vi "Link Control References.vi"(8 "error in":errorcluster, 10 "Control Map":T1[](array[typedef]), 11 "DIG_IO in":refnum<class "DIG_IO.lvclass">) -> (0 "error out":errorcluster, 3 "DIG_IO out":refnum<class "DIG_IO.lvclass">)   [LabVIEW 2019, in "DIG_IO.lvlib" / "DIG_IO.lvclass"]
uses:
  Library/DIG_IO.lvclass
  builds/Instruments/Instruments.lvlibp/Custom Controls/Control Element.ctl
  Library/DIG_IO.lvclass/DIG_IO.ctl
  builds/Instruments/Instruments.lvlibp/Library/Instruments.lvclass
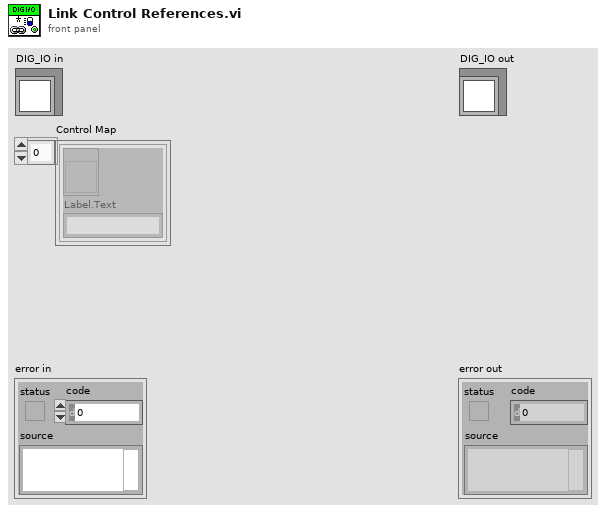
[diagram p1: front panel]
types:
  T1 = typedef "Instruments.lvlibp/Instruments.lvclass/Control Element.ctl" = cluster{refnum<vi>, "Label.Text":string}
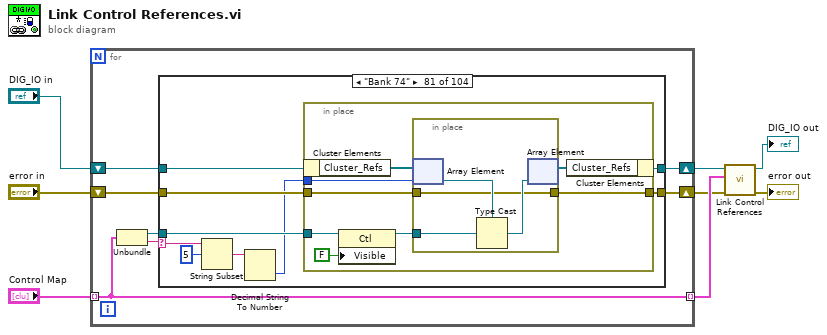
[diagram p0: block diagram]
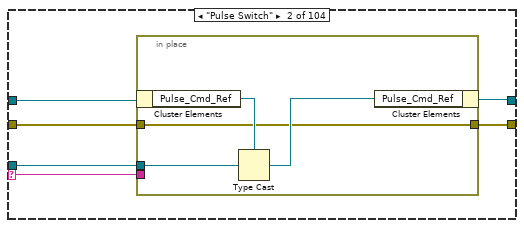
[diagram p3: hidden frame]
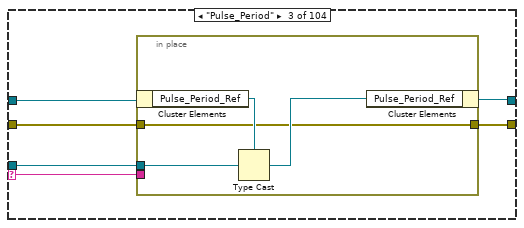
[diagram p4: hidden frame]
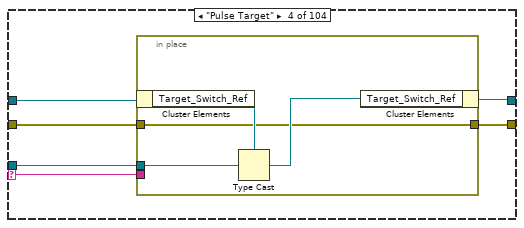
[diagram p5: hidden frame]
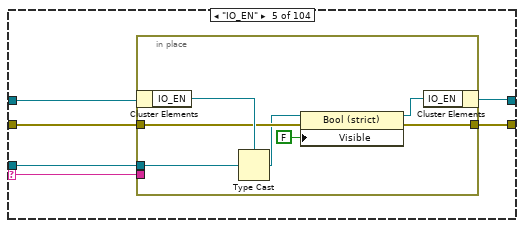
[diagram p6: hidden frame]
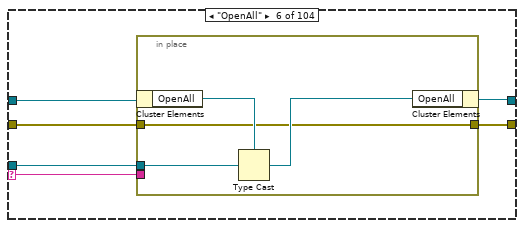
[diagram p7: hidden frame]
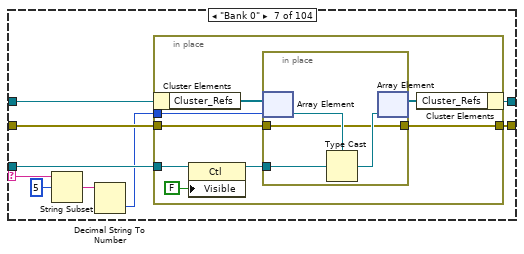
[diagram p8: hidden frame]
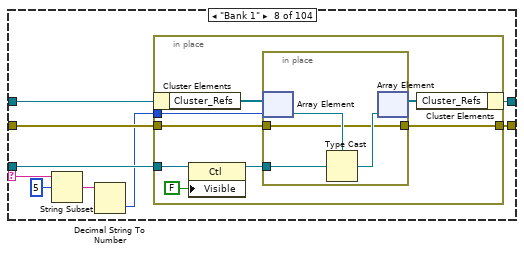
[diagram p9: hidden frame]
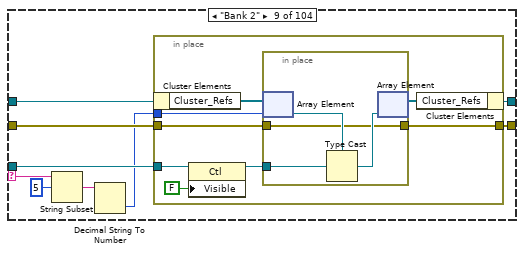
[diagram p10: hidden frame]
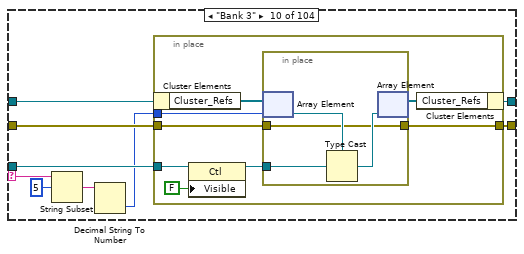
[diagram p11: hidden frame]
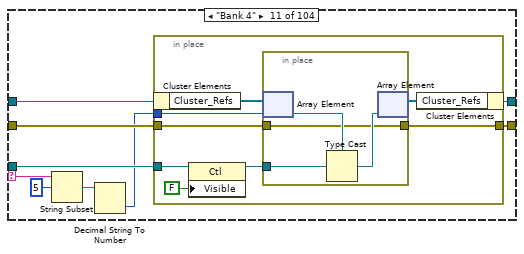
[diagram p12: hidden frame]
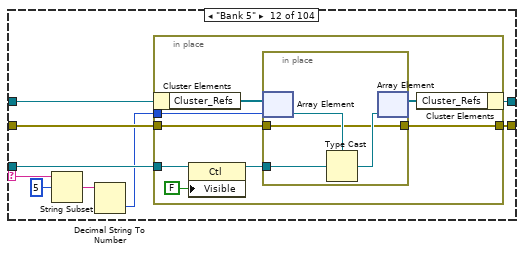
[diagram p13: hidden frame]
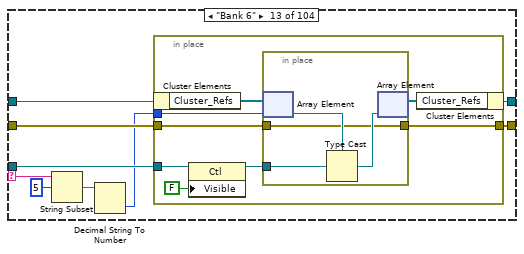
[diagram p14: hidden frame]
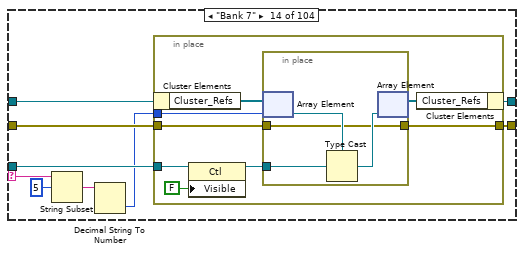
[diagram p15: hidden frame]
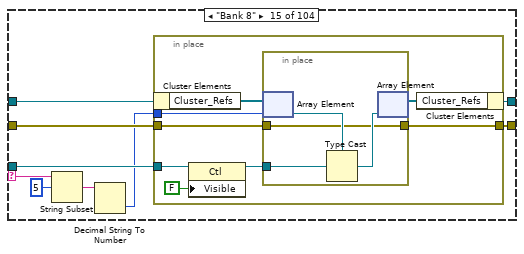
[diagram p16: hidden frame]
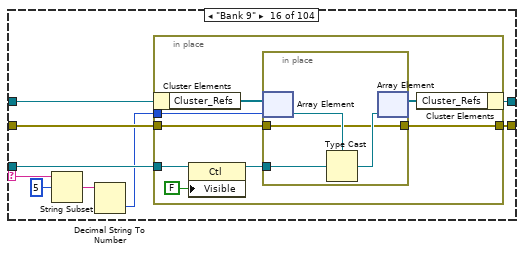
[diagram p17: hidden frame]
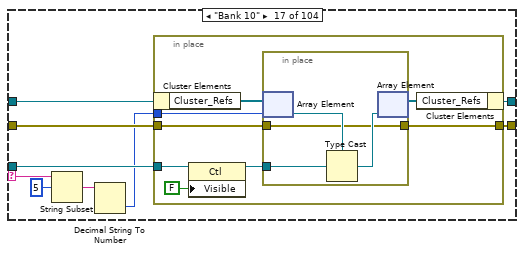
[diagram p18: hidden frame]
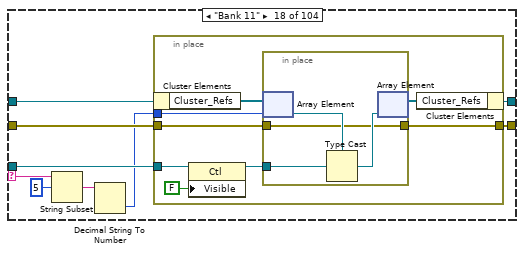
[diagram p19: hidden frame]
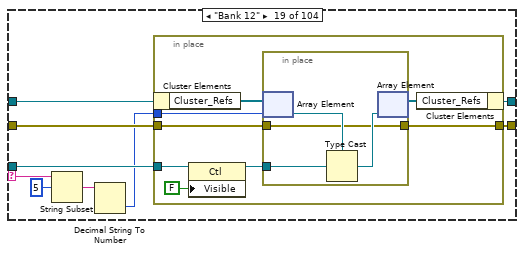
[diagram p20: hidden frame]
diagram:
  n1 = for {
    tunnel: "Control Map" -> [w15] mode=indexing
    tunnel: [w15] -> w5 mode=indexing
    shift-right: [w9] -> w3
    shift-left: "error in" -> [w12]
    shift-right: [w10] -> w1
    shift-left: "DIG_IO in" -> [w11]
    n2 = Unbundle(w15) -> (w13:refnum<vi>, "Label.Text"=w14:string)
    n3 = case shown="\"Bank 74\"" w14 {
      selector: w14 -> [_ w19 w29 w39 w49 w62 w72 w93 w114 w135 w156 w177 w198 w219 w240 w261 w282 w303 w324 w345 w366 w387 w408 w429 w450 w471 w492 w513 w534 w555 w576 w597 w618 w639 w660 w681 w702 w723 w744 w765 w786 w807 w828 w849 w870 w891 w912 w933 w954 w975 w996 w1017 w1038 w1059 w1080 w1101 w1122 w1143 w1164 w1185 w1206 w1227 w1248 w1269 w1290 w1311 w1332 w1353 w1374 w1395 w1416 w1437 w1458 w1479 w1500 w1521 w1542 w1563 w1584 w1605 w1626 w1647 w1668 w1689 w1710 w1731 w1752 w1773 w1794 w1815 w1836 w1857 w1878 w1899 w1920 w1941 w1962 w1983 w2004 w2025 w2046 w2067 w2088 w2103]
      tunnel: w13 -> [_ w20 w30 w40 w50 w63 w76 w97 w118 w139 w160 w181 w202 w223 w244 w265 w286 w307 w328 w349 w370 w391 w412 w433 w454 w475 w496 w517 w538 w559 w580 w601 w622 w643 w664 w685 w706 w727 w748 w769 w790 w811 w832 w853 w874 w895 w916 w937 w958 w979 w1000 w1021 w1042 w1063 w1084 w1105 w1126 w1147 w1168 w1189 w1210 w1231 w1252 w1273 w1294 w1315 w1336 w1357 w1378 w1399 w1420 w1441 w1462 w1483 w1504 w1525 w1546 w1567 w1588 w1609 w1630 w1651 w1672 w1693 w1714 w1735 w1756 w1777 w1798 w1819 w1840 w1861 w1882 w1903 w1924 w1945 w1966 w1987 w2008 w2029 w2050 w2071 w2092 w2107]
      tunnel: w12 -> [w16 w22 w32 w42 w52 w65 w78 w99 w120 w141 w162 w183 w204 w225 w246 w267 w288 w309 w330 w351 w372 w393 w414 w435 w456 w477 w498 w519 w540 w561 w582 w603 w624 w645 w666 w687 w708 w729 w750 w771 w792 w813 w834 w855 w876 w897 w918 w939 w960 w981 w1002 w1023 w1044 w1065 w1086 w1107 w1128 w1149 w1170 w1191 w1212 w1233 w1254 w1275 w1296 w1317 w1338 w1359 w1380 w1401 w1422 w1443 w1464 w1485 w1506 w1527 w1548 w1569 w1590 w1611 w1632 w1653 w1674 w1695 w1716 w1737 w1758 w1779 w1800 w1821 w1842 w1863 w1884 w1905 w1926 w1947 w1968 w1989 w2010 w2031 w2052 w2073 w2094 w2109]
      tunnel: w11 -> [w17 w23 w33 w43 w53 w66 w79 w100 w121 w142 w163 w184 w205 w226 w247 w268 w289 w310 w331 w352 w373 w394 w415 w436 w457 w478 w499 w520 w541 w562 w583 w604 w625 w646 w667 w688 w709 w730 w751 w772 w793 w814 w835 w856 w877 w898 w919 w940 w961 w982 w1003 w1024 w1045 w1066 w1087 w1108 w1129 w1150 w1171 w1192 w1213 w1234 w1255 w1276 w1297 w1318 w1339 w1360 w1381 w1402 w1423 w1444 w1465 w1486 w1507 w1528 w1549 w1570 w1591 w1612 w1633 w1654 w1675 w1696 w1717 w1738 w1759 w1780 w1801 w1822 w1843 w1864 w1885 w1906 w1927 w1948 w1969 w1990 w2011 w2032 w2053 w2074 w2095 w2110]
      tunnel: [w17 w21 w31 w41 w51 w64 w77 w98 w119 w140 w161 w182 w203 w224 w245 w266 w287 w308 w329 w350 w371 w392 w413 w434 w455 w476 w497 w518 w539 w560 w581 w602 w623 w644 w665 w686 w707 w728 w749 w770 w791 w812 w833 w854 w875 w896 w917 w938 w959 w980 w1001 w1022 w1043 w1064 w1085 w1106 w1127 w1148 w1169 w1190 w1211 w1232 w1253 w1274 w1295 w1316 w1337 w1358 w1379 w1400 w1421 w1442 w1463 w1484 w1505 w1526 w1547 w1568 w1589 w1610 w1631 w1652 w1673 w1694 w1715 w1736 w1757 w1778 w1799 w1820 w1841 w1862 w1883 w1904 w1925 w1946 w1967 w1988 w2009 w2030 w2051 w2072 w2093 w2108] -> w10
      tunnel: [w16 w18 w28 w38 w48 w61 w75 w96 w117 w138 w159 w180 w201 w222 w243 w264 w285 w306 w327 w348 w369 w390 w411 w432 w453 w474 w495 w516 w537 w558 w579 w600 w621 w642 w663 w684 w705 w726 w747 w768 w789 w810 w831 w852 w873 w894 w915 w936 w957 w978 w999 w1020 w1041 w1062 w1083 w1104 w1125 w1146 w1167 w1188 w1209 w1230 w1251 w1272 w1293 w1314 w1335 w1356 w1377 w1398 w1419 w1440 w1461 w1482 w1503 w1524 w1545 w1566 w1587 w1608 w1629 w1650 w1671 w1692 w1713 w1734 w1755 w1776 w1797 w1818 w1839 w1860 w1881 w1902 w1923 w1944 w1965 w1986 w2007 w2028 w2049 w2070 w2091 w2106] -> w9
      frame Default {
      }
      frame "Pulse Switch" {
        n4 = in-place {
          in-place-border: w22 -> [w24]
          in-place-border: w20 -> [w26]
          in-place-border: w19 -> [_]
          in-place-border: [w24] -> w18
          n5 = in-place-cluster #1(w23) -> ("Pulse_Cmd_Ref"=w27:refnum<vi>)
          n6 = Type Cast(type=w27, x=w26) -> (*(type *) &x=w25:refnum<vi>)
          n7 = in-place-cluster #1("Pulse_Cmd_Ref"=w25) -> (w21:refnum<class "DIG_IO.lvclass">)
        }
      }
      frame "Pulse_Period" {
        n8 = in-place {
          in-place-border: w32 -> [w34]
          in-place-border: w30 -> [w36]
          in-place-border: w29 -> [_]
          in-place-border: [w34] -> w28
          n9 = in-place-cluster #2(w33) -> ("Pulse_Period_Ref"=w37:refnum<vi>)
          n10 = Type Cast(type=w37, x=w36) -> (*(type *) &x=w35:refnum<vi>)
          n11 = in-place-cluster #2("Pulse_Period_Ref"=w35) -> (w31:refnum<class "DIG_IO.lvclass">)
        }
      }
      frame "Pulse Target" {
        n12 = in-place {
          in-place-border: w42 -> [w44]
          in-place-border: w40 -> [w46]
          in-place-border: w39 -> [_]
          in-place-border: [w44] -> w38
          n13 = in-place-cluster #3(w43) -> ("Target_Switch_Ref"=w47:refnum<vi>)
          n14 = Type Cast(type=w47, x=w46) -> (*(type *) &x=w45:refnum<vi>)
          n15 = in-place-cluster #3("Target_Switch_Ref"=w45) -> (w41:refnum<class "DIG_IO.lvclass">)
        }
      }
      frame "IO_EN" {
        n16 = in-place {
          in-place-border: w52 -> [w58]
          in-place-border: w50 -> [w59]
          in-place-border: w49 -> [_]
          in-place-border: [w57] -> w48
          n17 = in-place-cluster #4(w53) -> ("IO_EN"=w60:refnum<vi>)
          n18 = Type Cast(type=w60, x=w59) -> (*(type *) &x=w56:refnum<vi>)
          n19 = property class="Bool (strict)"(reference=w56, error in=w58, "Visible"=FALSE) -> (reference out=w55:refnum<vi>, error out=w57:errorcluster)
          n20 = in-place-cluster #4("IO_EN"=w55) -> (w51:refnum<class "DIG_IO.lvclass">)
        }
      }
      frame "OpenAll" {
        n21 = in-place {
          in-place-border: w65 -> [w67]
          in-place-border: w63 -> [w69]
          in-place-border: w62 -> [_]
          in-place-border: [w67] -> w61
          n22 = in-place-cluster #5(w66) -> ("OpenAll"=w70:refnum<vi>)
          n23 = Type Cast(type=w70, x=w69) -> (*(type *) &x=w68:refnum<vi>)
          n24 = in-place-cluster #5("OpenAll"=w68) -> (w64:refnum<class "DIG_IO.lvclass">)
        }
      }
      frame "Bank 0" {
        n25 = String Subset(string=w72, offset (0)=5) -> (substring=w74:string)  [unwired: 1 in]
        n26 = Decimal String To Number(string=w74) -> (number=w71:i32)  [unwired: 2 in, 1 out]
        n27 = in-place {
          in-place-border: w78 -> [w84]
          in-place-border: w76 -> [w85]
          in-place-border: [w83] -> w75
          in-place-border: w71 -> [w82]
          n28 = in-place-cluster #6(w79) -> ("Cluster_Refs"=w87:refnum<vi>[])
          n29 = property class="Ctl"(reference=w85, "Visible"=FALSE) -> (reference out=w81:refnum<vi>)  [unwired: 1 in, 1 out]
          n30 = in-place {
            in-place-border: w81 -> [w90]
            in-place-border: w84 -> [w88]
            in-place-border: [w88] -> w83
            n31 = in-place-array #7(w87, w82) -> (w91:refnum<vi>)
            n32 = Type Cast(type=w91, x=w90) -> (*(type *) &x=w89:refnum<vi>)
            n33 = in-place-array #7(w89) -> (w86:refnum<vi>[])  [unwired: 1 out]
          }
          n34 = in-place-cluster #6("Cluster_Refs"=w86) -> (w77:refnum<class "DIG_IO.lvclass">)
        }
      }
      frame "Bank 1" {
        n35 = String Subset(string=w93, offset (0)=5) -> (substring=w95:string)  [unwired: 1 in]
        n36 = Decimal String To Number(string=w95) -> (number=w92:i32)  [unwired: 2 in, 1 out]
        n37 = in-place {
          in-place-border: w99 -> [w105]
          in-place-border: w97 -> [w106]
          in-place-border: [w104] -> w96
          in-place-border: w92 -> [w103]
          n38 = in-place-cluster #8(w100) -> ("Cluster_Refs"=w108:refnum<vi>[])
          n39 = property class="Ctl"(reference=w106, "Visible"=FALSE) -> (reference out=w102:refnum<vi>)  [unwired: 1 in, 1 out]
          n40 = in-place {
            in-place-border: w102 -> [w111]
            in-place-border: w105 -> [w109]
            in-place-border: [w109] -> w104
            n41 = in-place-array #9(w108, w103) -> (w112:refnum<vi>)
            n42 = Type Cast(type=w112, x=w111) -> (*(type *) &x=w110:refnum<vi>)
            n43 = in-place-array #9(w110) -> (w107:refnum<vi>[])  [unwired: 1 out]
          }
          n44 = in-place-cluster #8("Cluster_Refs"=w107) -> (w98:refnum<class "DIG_IO.lvclass">)
        }
      }
      frame "Bank 2" {
        n45 = String Subset(string=w114, offset (0)=5) -> (substring=w116:string)  [unwired: 1 in]
        n46 = Decimal String To Number(string=w116) -> (number=w113:i32)  [unwired: 2 in, 1 out]
        n47 = in-place {
          in-place-border: w120 -> [w126]
          in-place-border: w118 -> [w127]
          in-place-border: [w125] -> w117
          in-place-border: w113 -> [w124]
          n48 = in-place-cluster #10(w121) -> ("Cluster_Refs"=w129:refnum<vi>[])
          n49 = property class="Ctl"(reference=w127, "Visible"=FALSE) -> (reference out=w123:refnum<vi>)  [unwired: 1 in, 1 out]
          n50 = in-place {
            in-place-border: w123 -> [w132]
            in-place-border: w126 -> [w130]
            in-place-border: [w130] -> w125
            n51 = in-place-array #11(w129, w124) -> (w133:refnum<vi>)
            n52 = Type Cast(type=w133, x=w132) -> (*(type *) &x=w131:refnum<vi>)
            n53 = in-place-array #11(w131) -> (w128:refnum<vi>[])  [unwired: 1 out]
          }
          n54 = in-place-cluster #10("Cluster_Refs"=w128) -> (w119:refnum<class "DIG_IO.lvclass">)
        }
      }
      frame "Bank 3" {
        n55 = String Subset(string=w135, offset (0)=5) -> (substring=w137:string)  [unwired: 1 in]
        n56 = Decimal String To Number(string=w137) -> (number=w134:i32)  [unwired: 2 in, 1 out]
        n57 = in-place {
          in-place-border: w141 -> [w147]
          in-place-border: w139 -> [w148]
          in-place-border: [w146] -> w138
          in-place-border: w134 -> [w145]
          n58 = in-place-cluster #12(w142) -> ("Cluster_Refs"=w150:refnum<vi>[])
          n59 = property class="Ctl"(reference=w148, "Visible"=FALSE) -> (reference out=w144:refnum<vi>)  [unwired: 1 in, 1 out]
          n60 = in-place {
            in-place-border: w144 -> [w153]
            in-place-border: w147 -> [w151]
            in-place-border: [w151] -> w146
            n61 = in-place-array #13(w150, w145) -> (w154:refnum<vi>)
            n62 = Type Cast(type=w154, x=w153) -> (*(type *) &x=w152:refnum<vi>)
            n63 = in-place-array #13(w152) -> (w149:refnum<vi>[])  [unwired: 1 out]
          }
          n64 = in-place-cluster #12("Cluster_Refs"=w149) -> (w140:refnum<class "DIG_IO.lvclass">)
        }
      }
      frame "Bank 4" {
        n65 = String Subset(string=w156, offset (0)=5) -> (substring=w158:string)  [unwired: 1 in]
        n66 = Decimal String To Number(string=w158) -> (number=w155:i32)  [unwired: 2 in, 1 out]
        n67 = in-place {
          in-place-border: w162 -> [w168]
          in-place-border: w160 -> [w169]
          in-place-border: [w167] -> w159
          in-place-border: w155 -> [w166]
          n68 = in-place-cluster #14(w163) -> ("Cluster_Refs"=w171:refnum<vi>[])
          n69 = property class="Ctl"(reference=w169, "Visible"=FALSE) -> (reference out=w165:refnum<vi>)  [unwired: 1 in, 1 out]
          n70 = in-place {
            in-place-border: w165 -> [w174]
            in-place-border: w168 -> [w172]
            in-place-border: [w172] -> w167
            n71 = in-place-array #15(w171, w166) -> (w175:refnum<vi>)
            n72 = Type Cast(type=w175, x=w174) -> (*(type *) &x=w173:refnum<vi>)
            n73 = in-place-array #15(w173) -> (w170:refnum<vi>[])  [unwired: 1 out]
          }
          n74 = in-place-cluster #14("Cluster_Refs"=w170) -> (w161:refnum<class "DIG_IO.lvclass">)
        }
      }
      frame "Bank 5" {
        n75 = String Subset(string=w177, offset (0)=5) -> (substring=w179:string)  [unwired: 1 in]
        n76 = Decimal String To Number(string=w179) -> (number=w176:i32)  [unwired: 2 in, 1 out]
        n77 = in-place {
          in-place-border: w183 -> [w189]
          in-place-border: w181 -> [w190]
          in-place-border: [w188] -> w180
          in-place-border: w176 -> [w187]
          n78 = in-place-cluster #16(w184) -> ("Cluster_Refs"=w192:refnum<vi>[])
          n79 = property class="Ctl"(reference=w190, "Visible"=FALSE) -> (reference out=w186:refnum<vi>)  [unwired: 1 in, 1 out]
          n80 = in-place {
            in-place-border: w186 -> [w195]
            in-place-border: w189 -> [w193]
            in-place-border: [w193] -> w188
            n81 = in-place-array #17(w192, w187) -> (w196:refnum<vi>)
            n82 = Type Cast(type=w196, x=w195) -> (*(type *) &x=w194:refnum<vi>)
            n83 = in-place-array #17(w194) -> (w191:refnum<vi>[])  [unwired: 1 out]
          }
          n84 = in-place-cluster #16("Cluster_Refs"=w191) -> (w182:refnum<class "DIG_IO.lvclass">)
        }
      }
      frame "Bank 6" {
        n85 = String Subset(string=w198, offset (0)=5) -> (substring=w200:string)  [unwired: 1 in]
        n86 = Decimal String To Number(string=w200) -> (number=w197:i32)  [unwired: 2 in, 1 out]
        n87 = in-place {
          in-place-border: w204 -> [w210]
          in-place-border: w202 -> [w211]
          in-place-border: [w209] -> w201
          in-place-border: w197 -> [w208]
          n88 = in-place-cluster #18(w205) -> ("Cluster_Refs"=w213:refnum<vi>[])
          n89 = property class="Ctl"(reference=w211, "Visible"=FALSE) -> (reference out=w207:refnum<vi>)  [unwired: 1 in, 1 out]
          n90 = in-place {
            in-place-border: w207 -> [w216]
            in-place-border: w210 -> [w214]
            in-place-border: [w214] -> w209
            n91 = in-place-array #19(w213, w208) -> (w217:refnum<vi>)
            n92 = Type Cast(type=w217, x=w216) -> (*(type *) &x=w215:refnum<vi>)
            n93 = in-place-array #19(w215) -> (w212:refnum<vi>[])  [unwired: 1 out]
          }
          n94 = in-place-cluster #18("Cluster_Refs"=w212) -> (w203:refnum<class "DIG_IO.lvclass">)
        }
      }
      frame "Bank 7" {
        n95 = String Subset(string=w219, offset (0)=5) -> (substring=w221:string)  [unwired: 1 in]
        n96 = Decimal String To Number(string=w221) -> (number=w218:i32)  [unwired: 2 in, 1 out]
        n97 = in-place {
          in-place-border: w225 -> [w231]
          in-place-border: w223 -> [w232]
          in-place-border: [w230] -> w222
          in-place-border: w218 -> [w229]
          n98 = in-place-cluster #20(w226) -> ("Cluster_Refs"=w234:refnum<vi>[])
          n99 = property class="Ctl"(reference=w232, "Visible"=FALSE) -> (reference out=w228:refnum<vi>)  [unwired: 1 in, 1 out]
          n100 = in-place {
            in-place-border: w228 -> [w237]
            in-place-border: w231 -> [w235]
            in-place-border: [w235] -> w230
            n101 = in-place-array #21(w234, w229) -> (w238:refnum<vi>)
            n102 = Type Cast(type=w238, x=w237) -> (*(type *) &x=w236:refnum<vi>)
            n103 = in-place-array #21(w236) -> (w233:refnum<vi>[])  [unwired: 1 out]
          }
          n104 = in-place-cluster #20("Cluster_Refs"=w233) -> (w224:refnum<class "DIG_IO.lvclass">)
        }
      }
      frame "Bank 8" {
        n105 = String Subset(string=w240, offset (0)=5) -> (substring=w242:string)  [unwired: 1 in]
        n106 = Decimal String To Number(string=w242) -> (number=w239:i32)  [unwired: 2 in, 1 out]
        n107 = in-place {
          in-place-border: w246 -> [w252]
          in-place-border: w244 -> [w253]
          in-place-border: [w251] -> w243
          in-place-border: w239 -> [w250]
          n108 = in-place-cluster #22(w247) -> ("Cluster_Refs"=w255:refnum<vi>[])
          n109 = property class="Ctl"(reference=w253, "Visible"=FALSE) -> (reference out=w249:refnum<vi>)  [unwired: 1 in, 1 out]
          n110 = in-place {
            in-place-border: w249 -> [w258]
            in-place-border: w252 -> [w256]
            in-place-border: [w256] -> w251
            n111 = in-place-array #23(w255, w250) -> (w259:refnum<vi>)
            n112 = Type Cast(type=w259, x=w258) -> (*(type *) &x=w257:refnum<vi>)
            n113 = in-place-array #23(w257) -> (w254:refnum<vi>[])  [unwired: 1 out]
          }
          n114 = in-place-cluster #22("Cluster_Refs"=w254) -> (w245:refnum<class "DIG_IO.lvclass">)
        }
      }
      frame "Bank 9" {
        n115 = String Subset(string=w261, offset (0)=5) -> (substring=w263:string)  [unwired: 1 in]
        n116 = Decimal String To Number(string=w263) -> (number=w260:i32)  [unwired: 2 in, 1 out]
        n117 = in-place {
          in-place-border: w267 -> [w273]
          in-place-border: w265 -> [w274]
          in-place-border: [w272] -> w264
          in-place-border: w260 -> [w271]
          n118 = in-place-cluster #24(w268) -> ("Cluster_Refs"=w276:refnum<vi>[])
          n119 = property class="Ctl"(reference=w274, "Visible"=FALSE) -> (reference out=w270:refnum<vi>)  [unwired: 1 in, 1 out]
          n120 = in-place {
            in-place-border: w270 -> [w279]
            in-place-border: w273 -> [w277]
            in-place-border: [w277] -> w272
            n121 = in-place-array #25(w276, w271) -> (w280:refnum<vi>)
            n122 = Type Cast(type=w280, x=w279) -> (*(type *) &x=w278:refnum<vi>)
            n123 = in-place-array #25(w278) -> (w275:refnum<vi>[])  [unwired: 1 out]
          }
          n124 = in-place-cluster #24("Cluster_Refs"=w275) -> (w266:refnum<class "DIG_IO.lvclass">)
        }
      }
      frame "Bank 10" {
        n125 = String Subset(string=w282, offset (0)=5) -> (substring=w284:string)  [unwired: 1 in]
        n126 = Decimal String To Number(string=w284) -> (number=w281:i32)  [unwired: 2 in, 1 out]
        n127 = in-place {
          in-place-border: w288 -> [w294]
          in-place-border: w286 -> [w295]
          in-place-border: [w293] -> w285
          in-place-border: w281 -> [w292]
          n128 = in-place-cluster #26(w289) -> ("Cluster_Refs"=w297:refnum<vi>[])
          n129 = property class="Ctl"(reference=w295, "Visible"=FALSE) -> (reference out=w291:refnum<vi>)  [unwired: 1 in, 1 out]
          n130 = in-place {
            in-place-border: w291 -> [w300]
            in-place-border: w294 -> [w298]
            in-place-border: [w298] -> w293
            n131 = in-place-array #27(w297, w292) -> (w301:refnum<vi>)
            n132 = Type Cast(type=w301, x=w300) -> (*(type *) &x=w299:refnum<vi>)
            n133 = in-place-array #27(w299) -> (w296:refnum<vi>[])  [unwired: 1 out]
          }
          n134 = in-place-cluster #26("Cluster_Refs"=w296) -> (w287:refnum<class "DIG_IO.lvclass">)
        }
      }
      frame "Bank 11" {
        n135 = String Subset(string=w303, offset (0)=5) -> (substring=w305:string)  [unwired: 1 in]
        n136 = Decimal String To Number(string=w305) -> (number=w302:i32)  [unwired: 2 in, 1 out]
        n137 = in-place {
          in-place-border: w309 -> [w315]
          in-place-border: w307 -> [w316]
          in-place-border: [w314] -> w306
          in-place-border: w302 -> [w313]
          n138 = in-place-cluster #28(w310) -> ("Cluster_Refs"=w318:refnum<vi>[])
          n139 = property class="Ctl"(reference=w316, "Visible"=FALSE) -> (reference out=w312:refnum<vi>)  [unwired: 1 in, 1 out]
          n140 = in-place {
            in-place-border: w312 -> [w321]
            in-place-border: w315 -> [w319]
            in-place-border: [w319] -> w314
            n141 = in-place-array #29(w318, w313) -> (w322:refnum<vi>)
            n142 = Type Cast(type=w322, x=w321) -> (*(type *) &x=w320:refnum<vi>)
            n143 = in-place-array #29(w320) -> (w317:refnum<vi>[])  [unwired: 1 out]
          }
          n144 = in-place-cluster #28("Cluster_Refs"=w317) -> (w308:refnum<class "DIG_IO.lvclass">)
        }
      }
      frame "Bank 12" {
        n145 = String Subset(string=w324, offset (0)=5) -> (substring=w326:string)  [unwired: 1 in]
        n146 = Decimal String To Number(string=w326) -> (number=w323:i32)  [unwired: 2 in, 1 out]
        n147 = in-place {
          in-place-border: w330 -> [w336]
          in-place-border: w328 -> [w337]
          in-place-border: [w335] -> w327
          in-place-border: w323 -> [w334]
          n148 = in-place-cluster #30(w331) -> ("Cluster_Refs"=w339:refnum<vi>[])
          n149 = property class="Ctl"(reference=w337, "Visible"=FALSE) -> (reference out=w333:refnum<vi>)  [unwired: 1 in, 1 out]
          n150 = in-place {
            in-place-border: w333 -> [w342]
            in-place-border: w336 -> [w340]
            in-place-border: [w340] -> w335
            n151 = in-place-array #31(w339, w334) -> (w343:refnum<vi>)
            n152 = Type Cast(type=w343, x=w342) -> (*(type *) &x=w341:refnum<vi>)
            n153 = in-place-array #31(w341) -> (w338:refnum<vi>[])  [unwired: 1 out]
          }
          n154 = in-place-cluster #30("Cluster_Refs"=w338) -> (w329:refnum<class "DIG_IO.lvclass">)
        }
      }
      frame "Bank 13" {
        n155 = String Subset(string=w345, offset (0)=5) -> (substring=w347:string)  [unwired: 1 in]
        n156 = Decimal String To Number(string=w347) -> (number=w344:i32)  [unwired: 2 in, 1 out]
        n157 = in-place {
          in-place-border: w351 -> [w357]
          in-place-border: w349 -> [w358]
          in-place-border: [w356] -> w348
          in-place-border: w344 -> [w355]
          n158 = in-place-cluster #32(w352) -> ("Cluster_Refs"=w360:refnum<vi>[])
          n159 = property class="Ctl"(reference=w358, "Visible"=FALSE) -> (reference out=w354:refnum<vi>)  [unwired: 1 in, 1 out]
          n160 = in-place {
            in-place-border: w354 -> [w363]
            in-place-border: w357 -> [w361]
            in-place-border: [w361] -> w356
            n161 = in-place-array #33(w360, w355) -> (w364:refnum<vi>)
            n162 = Type Cast(type=w364, x=w363) -> (*(type *) &x=w362:refnum<vi>)
            n163 = in-place-array #33(w362) -> (w359:refnum<vi>[])  [unwired: 1 out]
          }
          n164 = in-place-cluster #32("Cluster_Refs"=w359) -> (w350:refnum<class "DIG_IO.lvclass">)
        }
      }
      frame "Bank 14" {
        n165 = String Subset(string=w366, offset (0)=5) -> (substring=w368:string)  [unwired: 1 in]
        n166 = Decimal String To Number(string=w368) -> (number=w365:i32)  [unwired: 2 in, 1 out]
        n167 = in-place {
          in-place-border: w372 -> [w378]
          in-place-border: w370 -> [w379]
          in-place-border: [w377] -> w369
          in-place-border: w365 -> [w376]
          n168 = in-place-cluster #34(w373) -> ("Cluster_Refs"=w381:refnum<vi>[])
          n169 = property class="Ctl"(reference=w379, "Visible"=FALSE) -> (reference out=w375:refnum<vi>)  [unwired: 1 in, 1 out]
          n170 = in-place {
            in-place-border: w375 -> [w384]
            in-place-border: w378 -> [w382]
            in-place-border: [w382] -> w377
            n171 = in-place-array #35(w381, w376) -> (w385:refnum<vi>)
            n172 = Type Cast(type=w385, x=w384) -> (*(type *) &x=w383:refnum<vi>)
            n173 = in-place-array #35(w383) -> (w380:refnum<vi>[])  [unwired: 1 out]
          }
          n174 = in-place-cluster #34("Cluster_Refs"=w380) -> (w371:refnum<class "DIG_IO.lvclass">)
        }
      }
      frame "Bank 15" {
        n175 = String Subset(string=w387, offset (0)=5) -> (substring=w389:string)  [unwired: 1 in]
        n176 = Decimal String To Number(string=w389) -> (number=w386:i32)  [unwired: 2 in, 1 out]
        n177 = in-place {
          in-place-border: w393 -> [w399]
          in-place-border: w391 -> [w400]
          in-place-border: [w398] -> w390
          in-place-border: w386 -> [w397]
          n178 = in-place-cluster #36(w394) -> ("Cluster_Refs"=w402:refnum<vi>[])
          n179 = property class="Ctl"(reference=w400, "Visible"=FALSE) -> (reference out=w396:refnum<vi>)  [unwired: 1 in, 1 out]
          n180 = in-place {
            in-place-border: w396 -> [w405]
            in-place-border: w399 -> [w403]
            in-place-border: [w403] -> w398
            n181 = in-place-array #37(w402, w397) -> (w406:refnum<vi>)
            n182 = Type Cast(type=w406, x=w405) -> (*(type *) &x=w404:refnum<vi>)
            n183 = in-place-array #37(w404) -> (w401:refnum<vi>[])  [unwired: 1 out]
          }
          n184 = in-place-cluster #36("Cluster_Refs"=w401) -> (w392:refnum<class "DIG_IO.lvclass">)
        }
      }
      frame "Bank 16" {
        n185 = String Subset(string=w408, offset (0)=5) -> (substring=w410:string)  [unwired: 1 in]
        n186 = Decimal String To Number(string=w410) -> (number=w407:i32)  [unwired: 2 in, 1 out]
        n187 = in-place {
          in-place-border: w414 -> [w420]
          in-place-border: w412 -> [w421]
          in-place-border: [w419] -> w411
          in-place-border: w407 -> [w418]
          n188 = in-place-cluster #38(w415) -> ("Cluster_Refs"=w423:refnum<vi>[])
          n189 = property class="Ctl"(reference=w421, "Visible"=FALSE) -> (reference out=w417:refnum<vi>)  [unwired: 1 in, 1 out]
          n190 = in-place {
            in-place-border: w417 -> [w426]
            in-place-border: w420 -> [w424]
            in-place-border: [w424] -> w419
            n191 = in-place-array #39(w423, w418) -> (w427:refnum<vi>)
            n192 = Type Cast(type=w427, x=w426) -> (*(type *) &x=w425:refnum<vi>)
            n193 = in-place-array #39(w425) -> (w422:refnum<vi>[])  [unwired: 1 out]
          }
          n194 = in-place-cluster #38("Cluster_Refs"=w422) -> (w413:refnum<class "DIG_IO.lvclass">)
        }
      }
      frame "Bank 17" {
        n195 = String Subset(string=w429, offset (0)=5) -> (substring=w431:string)  [unwired: 1 in]
        n196 = Decimal String To Number(string=w431) -> (number=w428:i32)  [unwired: 2 in, 1 out]
        n197 = in-place {
          in-place-border: w435 -> [w441]
          in-place-border: w433 -> [w442]
          in-place-border: [w440] -> w432
          in-place-border: w428 -> [w439]
          n198 = in-place-cluster #40(w436) -> ("Cluster_Refs"=w444:refnum<vi>[])
          n199 = property class="Ctl"(reference=w442, "Visible"=FALSE) -> (reference out=w438:refnum<vi>)  [unwired: 1 in, 1 out]
          n200 = in-place {
            in-place-border: w438 -> [w447]
            in-place-border: w441 -> [w445]
            in-place-border: [w445] -> w440
            n201 = in-place-array #41(w444, w439) -> (w448:refnum<vi>)
            n202 = Type Cast(type=w448, x=w447) -> (*(type *) &x=w446:refnum<vi>)
            n203 = in-place-array #41(w446) -> (w443:refnum<vi>[])  [unwired: 1 out]
          }
          n204 = in-place-cluster #40("Cluster_Refs"=w443) -> (w434:refnum<class "DIG_IO.lvclass">)
        }
      }
      frame "Bank 18" {
        n205 = String Subset(string=w450, offset (0)=5) -> (substring=w452:string)  [unwired: 1 in]
        n206 = Decimal String To Number(string=w452) -> (number=w449:i32)  [unwired: 2 in, 1 out]
        n207 = in-place {
          in-place-border: w456 -> [w462]
          in-place-border: w454 -> [w463]
          in-place-border: [w461] -> w453
          in-place-border: w449 -> [w460]
          n208 = in-place-cluster #42(w457) -> ("Cluster_Refs"=w465:refnum<vi>[])
          n209 = property class="Ctl"(reference=w463, "Visible"=FALSE) -> (reference out=w459:refnum<vi>)  [unwired: 1 in, 1 out]
          n210 = in-place {
            in-place-border: w459 -> [w468]
            in-place-border: w462 -> [w466]
            in-place-border: [w466] -> w461
            n211 = in-place-array #43(w465, w460) -> (w469:refnum<vi>)
            n212 = Type Cast(type=w469, x=w468) -> (*(type *) &x=w467:refnum<vi>)
            n213 = in-place-array #43(w467) -> (w464:refnum<vi>[])  [unwired: 1 out]
          }
          n214 = in-place-cluster #42("Cluster_Refs"=w464) -> (w455:refnum<class "DIG_IO.lvclass">)
        }
      }
      frame "Bank 19" {
        n215 = String Subset(string=w471, offset (0)=5) -> (substring=w473:string)  [unwired: 1 in]
        n216 = Decimal String To Number(string=w473) -> (number=w470:i32)  [unwired: 2 in, 1 out]
        n217 = in-place {
          in-place-border: w477 -> [w483]
          in-place-border: w475 -> [w484]
          in-place-border: [w482] -> w474
          in-place-border: w470 -> [w481]
          n218 = in-place-cluster #44(w478) -> ("Cluster_Refs"=w486:refnum<vi>[])
          n219 = property class="Ctl"(reference=w484, "Visible"=FALSE) -> (reference out=w480:refnum<vi>)  [unwired: 1 in, 1 out]
          n220 = in-place {
            in-place-border: w480 -> [w489]
            in-place-border: w483 -> [w487]
            in-place-border: [w487] -> w482
            n221 = in-place-array #45(w486, w481) -> (w490:refnum<vi>)
            n222 = Type Cast(type=w490, x=w489) -> (*(type *) &x=w488:refnum<vi>)
            n223 = in-place-array #45(w488) -> (w485:refnum<vi>[])  [unwired: 1 out]
          }
          n224 = in-place-cluster #44("Cluster_Refs"=w485) -> (w476:refnum<class "DIG_IO.lvclass">)
        }
      }
      frame "Bank 20" {
        n225 = String Subset(string=w492, offset (0)=5) -> (substring=w494:string)  [unwired: 1 in]
        n226 = Decimal String To Number(string=w494) -> (number=w491:i32)  [unwired: 2 in, 1 out]
        n227 = in-place {
          in-place-border: w498 -> [w504]
          in-place-border: w496 -> [w505]
          in-place-border: [w503] -> w495
          in-place-border: w491 -> [w502]
          n228 = in-place-cluster #46(w499) -> ("Cluster_Refs"=w507:refnum<vi>[])
          n229 = property class="Ctl"(reference=w505, "Visible"=FALSE) -> (reference out=w501:refnum<vi>)  [unwired: 1 in, 1 out]
          n230 = in-place {
            in-place-border: w501 -> [w510]
            in-place-border: w504 -> [w508]
            in-place-border: [w508] -> w503
            n231 = in-place-array #47(w507, w502) -> (w511:refnum<vi>)
            n232 = Type Cast(type=w511, x=w510) -> (*(type *) &x=w509:refnum<vi>)
            n233 = in-place-array #47(w509) -> (w506:refnum<vi>[])  [unwired: 1 out]
          }
          n234 = in-place-cluster #46("Cluster_Refs"=w506) -> (w497:refnum<class "DIG_IO.lvclass">)
        }
      }
      frame "Bank 21" {
        n235 = String Subset(string=w513, offset (0)=5) -> (substring=w515:string)  [unwired: 1 in]
        n236 = Decimal String To Number(string=w515) -> (number=w512:i32)  [unwired: 2 in, 1 out]
        n237 = in-place {
          in-place-border: w519 -> [w525]
          in-place-border: w517 -> [w526]
          in-place-border: [w524] -> w516
          in-place-border: w512 -> [w523]
          n238 = in-place-cluster #48(w520) -> ("Cluster_Refs"=w528:refnum<vi>[])
          n239 = property class="Ctl"(reference=w526, "Visible"=FALSE) -> (reference out=w522:refnum<vi>)  [unwired: 1 in, 1 out]
          n240 = in-place {
            in-place-border: w522 -> [w531]
            in-place-border: w525 -> [w529]
            in-place-border: [w529] -> w524
            n241 = in-place-array #49(w528, w523) -> (w532:refnum<vi>)
            n242 = Type Cast(type=w532, x=w531) -> (*(type *) &x=w530:refnum<vi>)
            n243 = in-place-array #49(w530) -> (w527:refnum<vi>[])  [unwired: 1 out]
          }
          n244 = in-place-cluster #48("Cluster_Refs"=w527) -> (w518:refnum<class "DIG_IO.lvclass">)
        }
      }
      frame "Bank 22" {
        n245 = String Subset(string=w534, offset (0)=5) -> (substring=w536:string)  [unwired: 1 in]
        n246 = Decimal String To Number(string=w536) -> (number=w533:i32)  [unwired: 2 in, 1 out]
        n247 = in-place {
          in-place-border: w540 -> [w546]
          in-place-border: w538 -> [w547]
          in-place-border: [w545] -> w537
          in-place-border: w533 -> [w544]
          n248 = in-place-cluster #50(w541) -> ("Cluster_Refs"=w549:refnum<vi>[])
          n249 = property class="Ctl"(reference=w547, "Visible"=FALSE) -> (reference out=w543:refnum<vi>)  [unwired: 1 in, 1 out]
          n250 = in-place {
            in-place-border: w543 -> [w552]
            in-place-border: w546 -> [w550]
            in-place-border: [w550] -> w545
            n251 = in-place-array #51(w549, w544) -> (w553:refnum<vi>)
            n252 = Type Cast(type=w553, x=w552) -> (*(type *) &x=w551:refnum<vi>)
            n253 = in-place-array #51(w551) -> (w548:refnum<vi>[])  [unwired: 1 out]
          }
          n254 = in-place-cluster #50("Cluster_Refs"=w548) -> (w539:refnum<class "DIG_IO.lvclass">)
        }
      }
      frame "Bank 23" {
        n255 = String Subset(string=w555, offset (0)=5) -> (substring=w557:string)  [unwired: 1 in]
        n256 = Decimal String To Number(string=w557) -> (number=w554:i32)  [unwired: 2 in, 1 out]
        n257 = in-place {
          in-place-border: w561 -> [w567]
          in-place-border: w559 -> [w568]
          in-place-border: [w566] -> w558
          in-place-border: w554 -> [w565]
          n258 = in-place-cluster #52(w562) -> ("Cluster_Refs"=w570:refnum<vi>[])
          n259 = property class="Ctl"(reference=w568, "Visible"=FALSE) -> (reference out=w564:refnum<vi>)  [unwired: 1 in, 1 out]
          n260 = in-place {
            in-place-border: w564 -> [w573]
            in-place-border: w567 -> [w571]
            in-place-border: [w571] -> w566
            n261 = in-place-array #53(w570, w565) -> (w574:refnum<vi>)
            n262 = Type Cast(type=w574, x=w573) -> (*(type *) &x=w572:refnum<vi>)
            n263 = in-place-array #53(w572) -> (w569:refnum<vi>[])  [unwired: 1 out]
          }
          n264 = in-place-cluster #52("Cluster_Refs"=w569) -> (w560:refnum<class "DIG_IO.lvclass">)
        }
      }
      frame "Bank 24" {
        n265 = String Subset(string=w576, offset (0)=5) -> (substring=w578:string)  [unwired: 1 in]
        n266 = Decimal String To Number(string=w578) -> (number=w575:i32)  [unwired: 2 in, 1 out]
        n267 = in-place {
          in-place-border: w582 -> [w588]
          in-place-border: w580 -> [w589]
          in-place-border: [w587] -> w579
          in-place-border: w575 -> [w586]
          n268 = in-place-cluster #54(w583) -> ("Cluster_Refs"=w591:refnum<vi>[])
          n269 = property class="Ctl"(reference=w589, "Visible"=FALSE) -> (reference out=w585:refnum<vi>)  [unwired: 1 in, 1 out]
          n270 = in-place {
            in-place-border: w585 -> [w594]
            in-place-border: w588 -> [w592]
            in-place-border: [w592] -> w587
            n271 = in-place-array #55(w591, w586) -> (w595:refnum<vi>)
            n272 = Type Cast(type=w595, x=w594) -> (*(type *) &x=w593:refnum<vi>)
            n273 = in-place-array #55(w593) -> (w590:refnum<vi>[])  [unwired: 1 out]
          }
          n274 = in-place-cluster #54("Cluster_Refs"=w590) -> (w581:refnum<class "DIG_IO.lvclass">)
        }
      }
      frame "Bank 25" {
        n275 = String Subset(string=w597, offset (0)=5) -> (substring=w599:string)  [unwired: 1 in]
        n276 = Decimal String To Number(string=w599) -> (number=w596:i32)  [unwired: 2 in, 1 out]
        n277 = in-place {
          in-place-border: w603 -> [w609]
          in-place-border: w601 -> [w610]
          in-place-border: [w608] -> w600
          in-place-border: w596 -> [w607]
          n278 = in-place-cluster #56(w604) -> ("Cluster_Refs"=w612:refnum<vi>[])
          n279 = property class="Ctl"(reference=w610, "Visible"=FALSE) -> (reference out=w606:refnum<vi>)  [unwired: 1 in, 1 out]
          n280 = in-place {
            in-place-border: w606 -> [w615]
            in-place-border: w609 -> [w613]
            in-place-border: [w613] -> w608
            n281 = in-place-array #57(w612, w607) -> (w616:refnum<vi>)
            n282 = Type Cast(type=w616, x=w615) -> (*(type *) &x=w614:refnum<vi>)
            n283 = in-place-array #57(w614) -> (w611:refnum<vi>[])  [unwired: 1 out]
          }
          n284 = in-place-cluster #56("Cluster_Refs"=w611) -> (w602:refnum<class "DIG_IO.lvclass">)
        }
      }
      frame "Bank 26" {
        n285 = String Subset(string=w618, offset (0)=5) -> (substring=w620:string)  [unwired: 1 in]
        n286 = Decimal String To Number(string=w620) -> (number=w617:i32)  [unwired: 2 in, 1 out]
        n287 = in-place {
          in-place-border: w624 -> [w630]
          in-place-border: w622 -> [w631]
          in-place-border: [w629] -> w621
          in-place-border: w617 -> [w628]
          n288 = in-place-cluster #58(w625) -> ("Cluster_Refs"=w633:refnum<vi>[])
          n289 = property class="Ctl"(reference=w631, "Visible"=FALSE) -> (reference out=w627:refnum<vi>)  [unwired: 1 in, 1 out]
          n290 = in-place {
            in-place-border: w627 -> [w636]
            in-place-border: w630 -> [w634]
            in-place-border: [w634] -> w629
            n291 = in-place-array #59(w633, w628) -> (w637:refnum<vi>)
            n292 = Type Cast(type=w637, x=w636) -> (*(type *) &x=w635:refnum<vi>)
            n293 = in-place-array #59(w635) -> (w632:refnum<vi>[])  [unwired: 1 out]
          }
          n294 = in-place-cluster #58("Cluster_Refs"=w632) -> (w623:refnum<class "DIG_IO.lvclass">)
        }
      }
      frame "Bank 27" {
        n295 = String Subset(string=w639, offset (0)=5) -> (substring=w641:string)  [unwired: 1 in]
        n296 = Decimal String To Number(string=w641) -> (number=w638:i32)  [unwired: 2 in, 1 out]
        n297 = in-place {
          in-place-border: w645 -> [w651]
          in-place-border: w643 -> [w652]
          in-place-border: [w650] -> w642
          in-place-border: w638 -> [w649]
          n298 = in-place-cluster #60(w646) -> ("Cluster_Refs"=w654:refnum<vi>[])
          n299 = property class="Ctl"(reference=w652, "Visible"=FALSE) -> (reference out=w648:refnum<vi>)  [unwired: 1 in, 1 out]
          n300 = in-place {
            in-place-border: w648 -> [w657]
            in-place-border: w651 -> [w655]
            in-place-border: [w655] -> w650
            n301 = in-place-array #61(w654, w649) -> (w658:refnum<vi>)
            n302 = Type Cast(type=w658, x=w657) -> (*(type *) &x=w656:refnum<vi>)
            n303 = in-place-array #61(w656) -> (w653:refnum<vi>[])  [unwired: 1 out]
          }
          n304 = in-place-cluster #60("Cluster_Refs"=w653) -> (w644:refnum<class "DIG_IO.lvclass">)
        }
      }
      frame "Bank 28" {
        n305 = String Subset(string=w660, offset (0)=5) -> (substring=w662:string)  [unwired: 1 in]
        n306 = Decimal String To Number(string=w662) -> (number=w659:i32)  [unwired: 2 in, 1 out]
        n307 = in-place {
          in-place-border: w666 -> [w672]
          in-place-border: w664 -> [w673]
          in-place-border: [w671] -> w663
          in-place-border: w659 -> [w670]
          n308 = in-place-cluster #62(w667) -> ("Cluster_Refs"=w675:refnum<vi>[])
          n309 = property class="Ctl"(reference=w673, "Visible"=FALSE) -> (reference out=w669:refnum<vi>)  [unwired: 1 in, 1 out]
          n310 = in-place {
            in-place-border: w669 -> [w678]
            in-place-border: w672 -> [w676]
            in-place-border: [w676] -> w671
            n311 = in-place-array #63(w675, w670) -> (w679:refnum<vi>)
            n312 = Type Cast(type=w679, x=w678) -> (*(type *) &x=w677:refnum<vi>)
            n313 = in-place-array #63(w677) -> (w674:refnum<vi>[])  [unwired: 1 out]
          }
          n314 = in-place-cluster #62("Cluster_Refs"=w674) -> (w665:refnum<class "DIG_IO.lvclass">)
        }
      }
      frame "Bank 29" {
        n315 = String Subset(string=w681, offset (0)=5) -> (substring=w683:string)  [unwired: 1 in]
        n316 = Decimal String To Number(string=w683) -> (number=w680:i32)  [unwired: 2 in, 1 out]
        n317 = in-place {
          in-place-border: w687 -> [w693]
          in-place-border: w685 -> [w694]
          in-place-border: [w692] -> w684
          in-place-border: w680 -> [w691]
          n318 = in-place-cluster #64(w688) -> ("Cluster_Refs"=w696:refnum<vi>[])
          n319 = property class="Ctl"(reference=w694, "Visible"=FALSE) -> (reference out=w690:refnum<vi>)  [unwired: 1 in, 1 out]
          n320 = in-place {
            in-place-border: w690 -> [w699]
            in-place-border: w693 -> [w697]
            in-place-border: [w697] -> w692
            n321 = in-place-array #65(w696, w691) -> (w700:refnum<vi>)
            n322 = Type Cast(type=w700, x=w699) -> (*(type *) &x=w698:refnum<vi>)
            n323 = in-place-array #65(w698) -> (w695:refnum<vi>[])  [unwired: 1 out]
          }
          n324 = in-place-cluster #64("Cluster_Refs"=w695) -> (w686:refnum<class "DIG_IO.lvclass">)
        }
      }
      frame "Bank 30" {
        n325 = String Subset(string=w702, offset (0)=5) -> (substring=w704:string)  [unwired: 1 in]
        n326 = Decimal String To Number(string=w704) -> (number=w701:i32)  [unwired: 2 in, 1 out]
        n327 = in-place {
          in-place-border: w708 -> [w714]
          in-place-border: w706 -> [w715]
          in-place-border: [w713] -> w705
          in-place-border: w701 -> [w712]
          n328 = in-place-cluster #66(w709) -> ("Cluster_Refs"=w717:refnum<vi>[])
          n329 = property class="Ctl"(reference=w715, "Visible"=FALSE) -> (reference out=w711:refnum<vi>)  [unwired: 1 in, 1 out]
          n330 = in-place {
            in-place-border: w711 -> [w720]
            in-place-border: w714 -> [w718]
            in-place-border: [w718] -> w713
            n331 = in-place-array #67(w717, w712) -> (w721:refnum<vi>)
            n332 = Type Cast(type=w721, x=w720) -> (*(type *) &x=w719:refnum<vi>)
            n333 = in-place-array #67(w719) -> (w716:refnum<vi>[])  [unwired: 1 out]
          }
          n334 = in-place-cluster #66("Cluster_Refs"=w716) -> (w707:refnum<class "DIG_IO.lvclass">)
        }
      }
      frame "Bank 31" {
        n335 = String Subset(string=w723, offset (0)=5) -> (substring=w725:string)  [unwired: 1 in]
        n336 = Decimal String To Number(string=w725) -> (number=w722:i32)  [unwired: 2 in, 1 out]
        n337 = in-place {
          in-place-border: w729 -> [w735]
          in-place-border: w727 -> [w736]
          in-place-border: [w734] -> w726
          in-place-border: w722 -> [w733]
          n338 = in-place-cluster #68(w730) -> ("Cluster_Refs"=w738:refnum<vi>[])
          n339 = property class="Ctl"(reference=w736, "Visible"=FALSE) -> (reference out=w732:refnum<vi>)  [unwired: 1 in, 1 out]
          n340 = in-place {
            in-place-border: w732 -> [w741]
            in-place-border: w735 -> [w739]
            in-place-border: [w739] -> w734
            n341 = in-place-array #69(w738, w733) -> (w742:refnum<vi>)
            n342 = Type Cast(type=w742, x=w741) -> (*(type *) &x=w740:refnum<vi>)
            n343 = in-place-array #69(w740) -> (w737:refnum<vi>[])  [unwired: 1 out]
          }
          n344 = in-place-cluster #68("Cluster_Refs"=w737) -> (w728:refnum<class "DIG_IO.lvclass">)
        }
      }
      frame "Bank 32" {
        n345 = String Subset(string=w744, offset (0)=5) -> (substring=w746:string)  [unwired: 1 in]
        n346 = Decimal String To Number(string=w746) -> (number=w743:i32)  [unwired: 2 in, 1 out]
        n347 = in-place {
          in-place-border: w750 -> [w756]
          in-place-border: w748 -> [w757]
          in-place-border: [w755] -> w747
          in-place-border: w743 -> [w754]
          n348 = in-place-cluster #70(w751) -> ("Cluster_Refs"=w759:refnum<vi>[])
          n349 = property class="Ctl"(reference=w757, "Visible"=FALSE) -> (reference out=w753:refnum<vi>)  [unwired: 1 in, 1 out]
          n350 = in-place {
            in-place-border: w753 -> [w762]
            in-place-border: w756 -> [w760]
            in-place-border: [w760] -> w755
            n351 = in-place-array #71(w759, w754) -> (w763:refnum<vi>)
            n352 = Type Cast(type=w763, x=w762) -> (*(type *) &x=w761:refnum<vi>)
            n353 = in-place-array #71(w761) -> (w758:refnum<vi>[])  [unwired: 1 out]
          }
          n354 = in-place-cluster #70("Cluster_Refs"=w758) -> (w749:refnum<class "DIG_IO.lvclass">)
        }
      }
      frame "Bank 33" {
        n355 = String Subset(string=w765, offset (0)=5) -> (substring=w767:string)  [unwired: 1 in]
        n356 = Decimal String To Number(string=w767) -> (number=w764:i32)  [unwired: 2 in, 1 out]
        n357 = in-place {
          in-place-border: w771 -> [w777]
          in-place-border: w769 -> [w778]
          in-place-border: [w776] -> w768
          in-place-border: w764 -> [w775]
          n358 = in-place-cluster #72(w772) -> ("Cluster_Refs"=w780:refnum<vi>[])
          n359 = property class="Ctl"(reference=w778, "Visible"=FALSE) -> (reference out=w774:refnum<vi>)  [unwired: 1 in, 1 out]
          n360 = in-place {
            in-place-border: w774 -> [w783]
            in-place-border: w777 -> [w781]
            in-place-border: [w781] -> w776
            n361 = in-place-array #73(w780, w775) -> (w784:refnum<vi>)
            n362 = Type Cast(type=w784, x=w783) -> (*(type *) &x=w782:refnum<vi>)
            n363 = in-place-array #73(w782) -> (w779:refnum<vi>[])  [unwired: 1 out]
          }
          n364 = in-place-cluster #72("Cluster_Refs"=w779) -> (w770:refnum<class "DIG_IO.lvclass">)
        }
      }
      frame "Bank 34" {
        n365 = String Subset(string=w786, offset (0)=5) -> (substring=w788:string)  [unwired: 1 in]
        n366 = Decimal String To Number(string=w788) -> (number=w785:i32)  [unwired: 2 in, 1 out]
        n367 = in-place {
          in-place-border: w792 -> [w798]
          in-place-border: w790 -> [w799]
          in-place-border: [w797] -> w789
          in-place-border: w785 -> [w796]
          n368 = in-place-cluster #74(w793) -> ("Cluster_Refs"=w801:refnum<vi>[])
          n369 = property class="Ctl"(reference=w799, "Visible"=FALSE) -> (reference out=w795:refnum<vi>)  [unwired: 1 in, 1 out]
          n370 = in-place {
            in-place-border: w795 -> [w804]
            in-place-border: w798 -> [w802]
            in-place-border: [w802] -> w797
            n371 = in-place-array #75(w801, w796) -> (w805:refnum<vi>)
            n372 = Type Cast(type=w805, x=w804) -> (*(type *) &x=w803:refnum<vi>)
            n373 = in-place-array #75(w803) -> (w800:refnum<vi>[])  [unwired: 1 out]
          }
          n374 = in-place-cluster #74("Cluster_Refs"=w800) -> (w791:refnum<class "DIG_IO.lvclass">)
        }
      }
      frame "Bank 35" {
        n375 = String Subset(string=w807, offset (0)=5) -> (substring=w809:string)  [unwired: 1 in]
        n376 = Decimal String To Number(string=w809) -> (number=w806:i32)  [unwired: 2 in, 1 out]
        n377 = in-place {
          in-place-border: w813 -> [w819]
          in-place-border: w811 -> [w820]
          in-place-border: [w818] -> w810
          in-place-border: w806 -> [w817]
          n378 = in-place-cluster #76(w814) -> ("Cluster_Refs"=w822:refnum<vi>[])
          n379 = property class="Ctl"(reference=w820, "Visible"=FALSE) -> (reference out=w816:refnum<vi>)  [unwired: 1 in, 1 out]
          n380 = in-place {
            in-place-border: w816 -> [w825]
            in-place-border: w819 -> [w823]
            in-place-border: [w823] -> w818
            n381 = in-place-array #77(w822, w817) -> (w826:refnum<vi>)
            n382 = Type Cast(type=w826, x=w825) -> (*(type *) &x=w824:refnum<vi>)
            n383 = in-place-array #77(w824) -> (w821:refnum<vi>[])  [unwired: 1 out]
          }
          n384 = in-place-cluster #76("Cluster_Refs"=w821) -> (w812:refnum<class "DIG_IO.lvclass">)
        }
      }
      frame "Bank 36" {
        n385 = String Subset(string=w828, offset (0)=5) -> (substring=w830:string)  [unwired: 1 in]
        n386 = Decimal String To Number(string=w830) -> (number=w827:i32)  [unwired: 2 in, 1 out]
        n387 = in-place {
          in-place-border: w834 -> [w840]
          in-place-border: w832 -> [w841]
          in-place-border: [w839] -> w831
          in-place-border: w827 -> [w838]
          n388 = in-place-cluster #78(w835) -> ("Cluster_Refs"=w843:refnum<vi>[])
          n389 = property class="Ctl"(reference=w841, "Visible"=FALSE) -> (reference out=w837:refnum<vi>)  [unwired: 1 in, 1 out]
          n390 = in-place {
            in-place-border: w837 -> [w846]
            in-place-border: w840 -> [w844]
            in-place-border: [w844] -> w839
            n391 = in-place-array #79(w843, w838) -> (w847:refnum<vi>)
            n392 = Type Cast(type=w847, x=w846) -> (*(type *) &x=w845:refnum<vi>)
            n393 = in-place-array #79(w845) -> (w842:refnum<vi>[])  [unwired: 1 out]
          }
          n394 = in-place-cluster #78("Cluster_Refs"=w842) -> (w833:refnum<class "DIG_IO.lvclass">)
        }
      }
      frame "Bank 37" {
        n395 = String Subset(string=w849, offset (0)=5) -> (substring=w851:string)  [unwired: 1 in]
        n396 = Decimal String To Number(string=w851) -> (number=w848:i32)  [unwired: 2 in, 1 out]
        n397 = in-place {
          in-place-border: w855 -> [w861]
          in-place-border: w853 -> [w862]
          in-place-border: [w860] -> w852
          in-place-border: w848 -> [w859]
          n398 = in-place-cluster #80(w856) -> ("Cluster_Refs"=w864:refnum<vi>[])
          n399 = property class="Ctl"(reference=w862, "Visible"=FALSE) -> (reference out=w858:refnum<vi>)  [unwired: 1 in, 1 out]
          n400 = in-place {
            in-place-border: w858 -> [w867]
            in-place-border: w861 -> [w865]
            in-place-border: [w865] -> w860
            n401 = in-place-array #81(w864, w859) -> (w868:refnum<vi>)
            n402 = Type Cast(type=w868, x=w867) -> (*(type *) &x=w866:refnum<vi>)
            n403 = in-place-array #81(w866) -> (w863:refnum<vi>[])  [unwired: 1 out]
          }
          n404 = in-place-cluster #80("Cluster_Refs"=w863) -> (w854:refnum<class "DIG_IO.lvclass">)
        }
      }
      frame "Bank 38" {
        n405 = String Subset(string=w870, offset (0)=5) -> (substring=w872:string)  [unwired: 1 in]
        n406 = Decimal String To Number(string=w872) -> (number=w869:i32)  [unwired: 2 in, 1 out]
        n407 = in-place {
          in-place-border: w876 -> [w882]
          in-place-border: w874 -> [w883]
          in-place-border: [w881] -> w873
          in-place-border: w869 -> [w880]
          n408 = in-place-cluster #82(w877) -> ("Cluster_Refs"=w885:refnum<vi>[])
          n409 = property class="Ctl"(reference=w883, "Visible"=FALSE) -> (reference out=w879:refnum<vi>)  [unwired: 1 in, 1 out]
          n410 = in-place {
            in-place-border: w879 -> [w888]
            in-place-border: w882 -> [w886]
            in-place-border: [w886] -> w881
            n411 = in-place-array #83(w885, w880) -> (w889:refnum<vi>)
            n412 = Type Cast(type=w889, x=w888) -> (*(type *) &x=w887:refnum<vi>)
            n413 = in-place-array #83(w887) -> (w884:refnum<vi>[])  [unwired: 1 out]
          }
          n414 = in-place-cluster #82("Cluster_Refs"=w884) -> (w875:refnum<class "DIG_IO.lvclass">)
        }
      }
      frame "Bank 39" {
        n415 = String Subset(string=w891, offset (0)=5) -> (substring=w893:string)  [unwired: 1 in]
        n416 = Decimal String To Number(string=w893) -> (number=w890:i32)  [unwired: 2 in, 1 out]
        n417 = in-place {
          in-place-border: w897 -> [w903]
          in-place-border: w895 -> [w904]
          in-place-border: [w902] -> w894
          in-place-border: w890 -> [w901]
          n418 = in-place-cluster #84(w898) -> ("Cluster_Refs"=w906:refnum<vi>[])
          n419 = property class="Ctl"(reference=w904, "Visible"=FALSE) -> (reference out=w900:refnum<vi>)  [unwired: 1 in, 1 out]
          n420 = in-place {
            in-place-border: w900 -> [w909]
            in-place-border: w903 -> [w907]
            in-place-border: [w907] -> w902
            n421 = in-place-array #85(w906, w901) -> (w910:refnum<vi>)
            n422 = Type Cast(type=w910, x=w909) -> (*(type *) &x=w908:refnum<vi>)
            n423 = in-place-array #85(w908) -> (w905:refnum<vi>[])  [unwired: 1 out]
          }
          n424 = in-place-cluster #84("Cluster_Refs"=w905) -> (w896:refnum<class "DIG_IO.lvclass">)
        }
      }
      frame "Bank 40" {
        n425 = String Subset(string=w912, offset (0)=5) -> (substring=w914:string)  [unwired: 1 in]
        n426 = Decimal String To Number(string=w914) -> (number=w911:i32)  [unwired: 2 in, 1 out]
        n427 = in-place {
          in-place-border: w918 -> [w924]
          in-place-border: w916 -> [w925]
          in-place-border: [w923] -> w915
          in-place-border: w911 -> [w922]
          n428 = in-place-cluster #86(w919) -> ("Cluster_Refs"=w927:refnum<vi>[])
          n429 = property class="Ctl"(reference=w925, "Visible"=FALSE) -> (reference out=w921:refnum<vi>)  [unwired: 1 in, 1 out]
          n430 = in-place {
            in-place-border: w921 -> [w930]
            in-place-border: w924 -> [w928]
            in-place-border: [w928] -> w923
            n431 = in-place-array #87(w927, w922) -> (w931:refnum<vi>)
            n432 = Type Cast(type=w931, x=w930) -> (*(type *) &x=w929:refnum<vi>)
            n433 = in-place-array #87(w929) -> (w926:refnum<vi>[])  [unwired: 1 out]
          }
          n434 = in-place-cluster #86("Cluster_Refs"=w926) -> (w917:refnum<class "DIG_IO.lvclass">)
        }
      }
      frame "Bank 41" {
        n435 = String Subset(string=w933, offset (0)=5) -> (substring=w935:string)  [unwired: 1 in]
        n436 = Decimal String To Number(string=w935) -> (number=w932:i32)  [unwired: 2 in, 1 out]
        n437 = in-place {
          in-place-border: w939 -> [w945]
          in-place-border: w937 -> [w946]
          in-place-border: [w944] -> w936
          in-place-border: w932 -> [w943]
          n438 = in-place-cluster #88(w940) -> ("Cluster_Refs"=w948:refnum<vi>[])
          n439 = property class="Ctl"(reference=w946, "Visible"=FALSE) -> (reference out=w942:refnum<vi>)  [unwired: 1 in, 1 out]
          n440 = in-place {
            in-place-border: w942 -> [w951]
            in-place-border: w945 -> [w949]
            in-place-border: [w949] -> w944
            n441 = in-place-array #89(w948, w943) -> (w952:refnum<vi>)
            n442 = Type Cast(type=w952, x=w951) -> (*(type *) &x=w950:refnum<vi>)
            n443 = in-place-array #89(w950) -> (w947:refnum<vi>[])  [unwired: 1 out]
          }
          n444 = in-place-cluster #88("Cluster_Refs"=w947) -> (w938:refnum<class "DIG_IO.lvclass">)
        }
      }
      frame "Bank 42" {
        n445 = String Subset(string=w954, offset (0)=5) -> (substring=w956:string)  [unwired: 1 in]
        n446 = Decimal String To Number(string=w956) -> (number=w953:i32)  [unwired: 2 in, 1 out]
        n447 = in-place {
          in-place-border: w960 -> [w966]
          in-place-border: w958 -> [w967]
          in-place-border: [w965] -> w957
          in-place-border: w953 -> [w964]
          n448 = in-place-cluster #90(w961) -> ("Cluster_Refs"=w969:refnum<vi>[])
          n449 = property class="Ctl"(reference=w967, "Visible"=FALSE) -> (reference out=w963:refnum<vi>)  [unwired: 1 in, 1 out]
          n450 = in-place {
            in-place-border: w963 -> [w972]
            in-place-border: w966 -> [w970]
            in-place-border: [w970] -> w965
            n451 = in-place-array #91(w969, w964) -> (w973:refnum<vi>)
            n452 = Type Cast(type=w973, x=w972) -> (*(type *) &x=w971:refnum<vi>)
            n453 = in-place-array #91(w971) -> (w968:refnum<vi>[])  [unwired: 1 out]
          }
          n454 = in-place-cluster #90("Cluster_Refs"=w968) -> (w959:refnum<class "DIG_IO.lvclass">)
        }
      }
      frame "Bank 43" {
        n455 = String Subset(string=w975, offset (0)=5) -> (substring=w977:string)  [unwired: 1 in]
        n456 = Decimal String To Number(string=w977) -> (number=w974:i32)  [unwired: 2 in, 1 out]
        n457 = in-place {
          in-place-border: w981 -> [w987]
          in-place-border: w979 -> [w988]
          in-place-border: [w986] -> w978
          in-place-border: w974 -> [w985]
          n458 = in-place-cluster #92(w982) -> ("Cluster_Refs"=w990:refnum<vi>[])
          n459 = property class="Ctl"(reference=w988, "Visible"=FALSE) -> (reference out=w984:refnum<vi>)  [unwired: 1 in, 1 out]
          n460 = in-place {
            in-place-border: w984 -> [w993]
            in-place-border: w987 -> [w991]
            in-place-border: [w991] -> w986
            n461 = in-place-array #93(w990, w985) -> (w994:refnum<vi>)
            n462 = Type Cast(type=w994, x=w993) -> (*(type *) &x=w992:refnum<vi>)
            n463 = in-place-array #93(w992) -> (w989:refnum<vi>[])  [unwired: 1 out]
          }
          n464 = in-place-cluster #92("Cluster_Refs"=w989) -> (w980:refnum<class "DIG_IO.lvclass">)
        }
      }
      frame "Bank 44" {
        n465 = String Subset(string=w996, offset (0)=5) -> (substring=w998:string)  [unwired: 1 in]
        n466 = Decimal String To Number(string=w998) -> (number=w995:i32)  [unwired: 2 in, 1 out]
        n467 = in-place {
          in-place-border: w1002 -> [w1008]
          in-place-border: w1000 -> [w1009]
          in-place-border: [w1007] -> w999
          in-place-border: w995 -> [w1006]
          n468 = in-place-cluster #94(w1003) -> ("Cluster_Refs"=w1011:refnum<vi>[])
          n469 = property class="Ctl"(reference=w1009, "Visible"=FALSE) -> (reference out=w1005:refnum<vi>)  [unwired: 1 in, 1 out]
          n470 = in-place {
            in-place-border: w1005 -> [w1014]
            in-place-border: w1008 -> [w1012]
            in-place-border: [w1012] -> w1007
            n471 = in-place-array #95(w1011, w1006) -> (w1015:refnum<vi>)
            n472 = Type Cast(type=w1015, x=w1014) -> (*(type *) &x=w1013:refnum<vi>)
            n473 = in-place-array #95(w1013) -> (w1010:refnum<vi>[])  [unwired: 1 out]
          }
          n474 = in-place-cluster #94("Cluster_Refs"=w1010) -> (w1001:refnum<class "DIG_IO.lvclass">)
        }
      }
      frame "Bank 45" {
        n475 = String Subset(string=w1017, offset (0)=5) -> (substring=w1019:string)  [unwired: 1 in]
        n476 = Decimal String To Number(string=w1019) -> (number=w1016:i32)  [unwired: 2 in, 1 out]
        n477 = in-place {
          in-place-border: w1023 -> [w1029]
          in-place-border: w1021 -> [w1030]
          in-place-border: [w1028] -> w1020
          in-place-border: w1016 -> [w1027]
          n478 = in-place-cluster #96(w1024) -> ("Cluster_Refs"=w1032:refnum<vi>[])
          n479 = property class="Ctl"(reference=w1030, "Visible"=FALSE) -> (reference out=w1026:refnum<vi>)  [unwired: 1 in, 1 out]
          n480 = in-place {
            in-place-border: w1026 -> [w1035]
            in-place-border: w1029 -> [w1033]
            in-place-border: [w1033] -> w1028
            n481 = in-place-array #97(w1032, w1027) -> (w1036:refnum<vi>)
            n482 = Type Cast(type=w1036, x=w1035) -> (*(type *) &x=w1034:refnum<vi>)
            n483 = in-place-array #97(w1034) -> (w1031:refnum<vi>[])  [unwired: 1 out]
          }
          n484 = in-place-cluster #96("Cluster_Refs"=w1031) -> (w1022:refnum<class "DIG_IO.lvclass">)
        }
      }
      frame "Bank 46" {
        n485 = String Subset(string=w1038, offset (0)=5) -> (substring=w1040:string)  [unwired: 1 in]
        n486 = Decimal String To Number(string=w1040) -> (number=w1037:i32)  [unwired: 2 in, 1 out]
        n487 = in-place {
          in-place-border: w1044 -> [w1050]
          in-place-border: w1042 -> [w1051]
          in-place-border: [w1049] -> w1041
          in-place-border: w1037 -> [w1048]
          n488 = in-place-cluster #98(w1045) -> ("Cluster_Refs"=w1053:refnum<vi>[])
          n489 = property class="Ctl"(reference=w1051, "Visible"=FALSE) -> (reference out=w1047:refnum<vi>)  [unwired: 1 in, 1 out]
          n490 = in-place {
            in-place-border: w1047 -> [w1056]
            in-place-border: w1050 -> [w1054]
            in-place-border: [w1054] -> w1049
            n491 = in-place-array #99(w1053, w1048) -> (w1057:refnum<vi>)
            n492 = Type Cast(type=w1057, x=w1056) -> (*(type *) &x=w1055:refnum<vi>)
            n493 = in-place-array #99(w1055) -> (w1052:refnum<vi>[])  [unwired: 1 out]
          }
          n494 = in-place-cluster #98("Cluster_Refs"=w1052) -> (w1043:refnum<class "DIG_IO.lvclass">)
        }
      }
      frame "Bank 47" {
        n495 = String Subset(string=w1059, offset (0)=5) -> (substring=w1061:string)  [unwired: 1 in]
        n496 = Decimal String To Number(string=w1061) -> (number=w1058:i32)  [unwired: 2 in, 1 out]
        n497 = in-place {
          in-place-border: w1065 -> [w1071]
          in-place-border: w1063 -> [w1072]
          in-place-border: [w1070] -> w1062
          in-place-border: w1058 -> [w1069]
          n498 = in-place-cluster #100(w1066) -> ("Cluster_Refs"=w1074:refnum<vi>[])
          n499 = property class="Ctl"(reference=w1072, "Visible"=FALSE) -> (reference out=w1068:refnum<vi>)  [unwired: 1 in, 1 out]
          n500 = in-place {
            in-place-border: w1068 -> [w1077]
            in-place-border: w1071 -> [w1075]
            in-place-border: [w1075] -> w1070
            n501 = in-place-array #101(w1074, w1069) -> (w1078:refnum<vi>)
            n502 = Type Cast(type=w1078, x=w1077) -> (*(type *) &x=w1076:refnum<vi>)
            n503 = in-place-array #101(w1076) -> (w1073:refnum<vi>[])  [unwired: 1 out]
          }
          n504 = in-place-cluster #100("Cluster_Refs"=w1073) -> (w1064:refnum<class "DIG_IO.lvclass">)
        }
      }
      frame "Bank 48" {
        n505 = String Subset(string=w1080, offset (0)=5) -> (substring=w1082:string)  [unwired: 1 in]
        n506 = Decimal String To Number(string=w1082) -> (number=w1079:i32)  [unwired: 2 in, 1 out]
        n507 = in-place {
          in-place-border: w1086 -> [w1092]
          in-place-border: w1084 -> [w1093]
          in-place-border: [w1091] -> w1083
          in-place-border: w1079 -> [w1090]
          n508 = in-place-cluster #102(w1087) -> ("Cluster_Refs"=w1095:refnum<vi>[])
          n509 = property class="Ctl"(reference=w1093, "Visible"=FALSE) -> (reference out=w1089:refnum<vi>)  [unwired: 1 in, 1 out]
          n510 = in-place {
            in-place-border: w1089 -> [w1098]
            in-place-border: w1092 -> [w1096]
            in-place-border: [w1096] -> w1091
            n511 = in-place-array #103(w1095, w1090) -> (w1099:refnum<vi>)
            n512 = Type Cast(type=w1099, x=w1098) -> (*(type *) &x=w1097:refnum<vi>)
            n513 = in-place-array #103(w1097) -> (w1094:refnum<vi>[])  [unwired: 1 out]
          }
          n514 = in-place-cluster #102("Cluster_Refs"=w1094) -> (w1085:refnum<class "DIG_IO.lvclass">)
        }
      }
      frame "Bank 49" {
        n515 = String Subset(string=w1101, offset (0)=5) -> (substring=w1103:string)  [unwired: 1 in]
        n516 = Decimal String To Number(string=w1103) -> (number=w1100:i32)  [unwired: 2 in, 1 out]
        n517 = in-place {
          in-place-border: w1107 -> [w1113]
          in-place-border: w1105 -> [w1114]
          in-place-border: [w1112] -> w1104
          in-place-border: w1100 -> [w1111]
          n518 = in-place-cluster #104(w1108) -> ("Cluster_Refs"=w1116:refnum<vi>[])
          n519 = property class="Ctl"(reference=w1114, "Visible"=FALSE) -> (reference out=w1110:refnum<vi>)  [unwired: 1 in, 1 out]
          n520 = in-place {
            in-place-border: w1110 -> [w1119]
            in-place-border: w1113 -> [w1117]
            in-place-border: [w1117] -> w1112
            n521 = in-place-array #105(w1116, w1111) -> (w1120:refnum<vi>)
            n522 = Type Cast(type=w1120, x=w1119) -> (*(type *) &x=w1118:refnum<vi>)
            n523 = in-place-array #105(w1118) -> (w1115:refnum<vi>[])  [unwired: 1 out]
          }
          n524 = in-place-cluster #104("Cluster_Refs"=w1115) -> (w1106:refnum<class "DIG_IO.lvclass">)
        }
      }
      frame "Bank 50" {
        n525 = String Subset(string=w1122, offset (0)=5) -> (substring=w1124:string)  [unwired: 1 in]
        n526 = Decimal String To Number(string=w1124) -> (number=w1121:i32)  [unwired: 2 in, 1 out]
        n527 = in-place {
          in-place-border: w1128 -> [w1134]
          in-place-border: w1126 -> [w1135]
          in-place-border: [w1133] -> w1125
          in-place-border: w1121 -> [w1132]
          n528 = in-place-cluster #106(w1129) -> ("Cluster_Refs"=w1137:refnum<vi>[])
          n529 = property class="Ctl"(reference=w1135, "Visible"=FALSE) -> (reference out=w1131:refnum<vi>)  [unwired: 1 in, 1 out]
          n530 = in-place {
            in-place-border: w1131 -> [w1140]
            in-place-border: w1134 -> [w1138]
            in-place-border: [w1138] -> w1133
            n531 = in-place-array #107(w1137, w1132) -> (w1141:refnum<vi>)
            n532 = Type Cast(type=w1141, x=w1140) -> (*(type *) &x=w1139:refnum<vi>)
            n533 = in-place-array #107(w1139) -> (w1136:refnum<vi>[])  [unwired: 1 out]
          }
          n534 = in-place-cluster #106("Cluster_Refs"=w1136) -> (w1127:refnum<class "DIG_IO.lvclass">)
        }
      }
      frame "Bank 51" {
        n535 = String Subset(string=w1143, offset (0)=5) -> (substring=w1145:string)  [unwired: 1 in]
        n536 = Decimal String To Number(string=w1145) -> (number=w1142:i32)  [unwired: 2 in, 1 out]
        n537 = in-place {
          in-place-border: w1149 -> [w1155]
          in-place-border: w1147 -> [w1156]
          in-place-border: [w1154] -> w1146
          in-place-border: w1142 -> [w1153]
          n538 = in-place-cluster #108(w1150) -> ("Cluster_Refs"=w1158:refnum<vi>[])
          n539 = property class="Ctl"(reference=w1156, "Visible"=FALSE) -> (reference out=w1152:refnum<vi>)  [unwired: 1 in, 1 out]
          n540 = in-place {
            in-place-border: w1152 -> [w1161]
            in-place-border: w1155 -> [w1159]
            in-place-border: [w1159] -> w1154
            n541 = in-place-array #109(w1158, w1153) -> (w1162:refnum<vi>)
            n542 = Type Cast(type=w1162, x=w1161) -> (*(type *) &x=w1160:refnum<vi>)
            n543 = in-place-array #109(w1160) -> (w1157:refnum<vi>[])  [unwired: 1 out]
          }
          n544 = in-place-cluster #108("Cluster_Refs"=w1157) -> (w1148:refnum<class "DIG_IO.lvclass">)
        }
      }
      frame "Bank 52" {
        n545 = String Subset(string=w1164, offset (0)=5) -> (substring=w1166:string)  [unwired: 1 in]
        n546 = Decimal String To Number(string=w1166) -> (number=w1163:i32)  [unwired: 2 in, 1 out]
        n547 = in-place {
          in-place-border: w1170 -> [w1176]
          in-place-border: w1168 -> [w1177]
          in-place-border: [w1175] -> w1167
          in-place-border: w1163 -> [w1174]
          n548 = in-place-cluster #110(w1171) -> ("Cluster_Refs"=w1179:refnum<vi>[])
          n549 = property class="Ctl"(reference=w1177, "Visible"=FALSE) -> (reference out=w1173:refnum<vi>)  [unwired: 1 in, 1 out]
          n550 = in-place {
            in-place-border: w1173 -> [w1182]
            in-place-border: w1176 -> [w1180]
            in-place-border: [w1180] -> w1175
            n551 = in-place-array #111(w1179, w1174) -> (w1183:refnum<vi>)
            n552 = Type Cast(type=w1183, x=w1182) -> (*(type *) &x=w1181:refnum<vi>)
            n553 = in-place-array #111(w1181) -> (w1178:refnum<vi>[])  [unwired: 1 out]
          }
          n554 = in-place-cluster #110("Cluster_Refs"=w1178) -> (w1169:refnum<class "DIG_IO.lvclass">)
        }
      }
      frame "Bank 53" {
        n555 = String Subset(string=w1185, offset (0)=5) -> (substring=w1187:string)  [unwired: 1 in]
        n556 = Decimal String To Number(string=w1187) -> (number=w1184:i32)  [unwired: 2 in, 1 out]
        n557 = in-place {
          in-place-border: w1191 -> [w1197]
          in-place-border: w1189 -> [w1198]
          in-place-border: [w1196] -> w1188
          in-place-border: w1184 -> [w1195]
          n558 = in-place-cluster #112(w1192) -> ("Cluster_Refs"=w1200:refnum<vi>[])
          n559 = property class="Ctl"(reference=w1198, "Visible"=FALSE) -> (reference out=w1194:refnum<vi>)  [unwired: 1 in, 1 out]
          n560 = in-place {
            in-place-border: w1194 -> [w1203]
            in-place-border: w1197 -> [w1201]
            in-place-border: [w1201] -> w1196
            n561 = in-place-array #113(w1200, w1195) -> (w1204:refnum<vi>)
            n562 = Type Cast(type=w1204, x=w1203) -> (*(type *) &x=w1202:refnum<vi>)
            n563 = in-place-array #113(w1202) -> (w1199:refnum<vi>[])  [unwired: 1 out]
          }
          n564 = in-place-cluster #112("Cluster_Refs"=w1199) -> (w1190:refnum<class "DIG_IO.lvclass">)
        }
      }
      frame "Bank 54" {
        n565 = String Subset(string=w1206, offset (0)=5) -> (substring=w1208:string)  [unwired: 1 in]
        n566 = Decimal String To Number(string=w1208) -> (number=w1205:i32)  [unwired: 2 in, 1 out]
        n567 = in-place {
          in-place-border: w1212 -> [w1218]
          in-place-border: w1210 -> [w1219]
          in-place-border: [w1217] -> w1209
          in-place-border: w1205 -> [w1216]
          n568 = in-place-cluster #114(w1213) -> ("Cluster_Refs"=w1221:refnum<vi>[])
          n569 = property class="Ctl"(reference=w1219, "Visible"=FALSE) -> (reference out=w1215:refnum<vi>)  [unwired: 1 in, 1 out]
          n570 = in-place {
            in-place-border: w1215 -> [w1224]
            in-place-border: w1218 -> [w1222]
            in-place-border: [w1222] -> w1217
            n571 = in-place-array #115(w1221, w1216) -> (w1225:refnum<vi>)
            n572 = Type Cast(type=w1225, x=w1224) -> (*(type *) &x=w1223:refnum<vi>)
            n573 = in-place-array #115(w1223) -> (w1220:refnum<vi>[])  [unwired: 1 out]
          }
          n574 = in-place-cluster #114("Cluster_Refs"=w1220) -> (w1211:refnum<class "DIG_IO.lvclass">)
        }
      }
      frame "Bank 55" {
        n575 = String Subset(string=w1227, offset (0)=5) -> (substring=w1229:string)  [unwired: 1 in]
        n576 = Decimal String To Number(string=w1229) -> (number=w1226:i32)  [unwired: 2 in, 1 out]
        n577 = in-place {
          in-place-border: w1233 -> [w1239]
          in-place-border: w1231 -> [w1240]
          in-place-border: [w1238] -> w1230
          in-place-border: w1226 -> [w1237]
          n578 = in-place-cluster #116(w1234) -> ("Cluster_Refs"=w1242:refnum<vi>[])
          n579 = property class="Ctl"(reference=w1240, "Visible"=FALSE) -> (reference out=w1236:refnum<vi>)  [unwired: 1 in, 1 out]
          n580 = in-place {
            in-place-border: w1236 -> [w1245]
            in-place-border: w1239 -> [w1243]
            in-place-border: [w1243] -> w1238
            n581 = in-place-array #117(w1242, w1237) -> (w1246:refnum<vi>)
            n582 = Type Cast(type=w1246, x=w1245) -> (*(type *) &x=w1244:refnum<vi>)
            n583 = in-place-array #117(w1244) -> (w1241:refnum<vi>[])  [unwired: 1 out]
          }
          n584 = in-place-cluster #116("Cluster_Refs"=w1241) -> (w1232:refnum<class "DIG_IO.lvclass">)
        }
      }
      frame "Bank 56" {
        n585 = String Subset(string=w1248, offset (0)=5) -> (substring=w1250:string)  [unwired: 1 in]
        n586 = Decimal String To Number(string=w1250) -> (number=w1247:i32)  [unwired: 2 in, 1 out]
        n587 = in-place {
          in-place-border: w1254 -> [w1260]
          in-place-border: w1252 -> [w1261]
          in-place-border: [w1259] -> w1251
          in-place-border: w1247 -> [w1258]
          n588 = in-place-cluster #118(w1255) -> ("Cluster_Refs"=w1263:refnum<vi>[])
          n589 = property class="Ctl"(reference=w1261, "Visible"=FALSE) -> (reference out=w1257:refnum<vi>)  [unwired: 1 in, 1 out]
          n590 = in-place {
            in-place-border: w1257 -> [w1266]
            in-place-border: w1260 -> [w1264]
            in-place-border: [w1264] -> w1259
            n591 = in-place-array #119(w1263, w1258) -> (w1267:refnum<vi>)
            n592 = Type Cast(type=w1267, x=w1266) -> (*(type *) &x=w1265:refnum<vi>)
            n593 = in-place-array #119(w1265) -> (w1262:refnum<vi>[])  [unwired: 1 out]
          }
          n594 = in-place-cluster #118("Cluster_Refs"=w1262) -> (w1253:refnum<class "DIG_IO.lvclass">)
        }
      }
      frame "Bank 57" {
        n595 = String Subset(string=w1269, offset (0)=5) -> (substring=w1271:string)  [unwired: 1 in]
        n596 = Decimal String To Number(string=w1271) -> (number=w1268:i32)  [unwired: 2 in, 1 out]
        n597 = in-place {
          in-place-border: w1275 -> [w1281]
          in-place-border: w1273 -> [w1282]
          in-place-border: [w1280] -> w1272
          in-place-border: w1268 -> [w1279]
          n598 = in-place-cluster #120(w1276) -> ("Cluster_Refs"=w1284:refnum<vi>[])
          n599 = property class="Ctl"(reference=w1282, "Visible"=FALSE) -> (reference out=w1278:refnum<vi>)  [unwired: 1 in, 1 out]
          n600 = in-place {
            in-place-border: w1278 -> [w1287]
            in-place-border: w1281 -> [w1285]
            in-place-border: [w1285] -> w1280
            n601 = in-place-array #121(w1284, w1279) -> (w1288:refnum<vi>)
            n602 = Type Cast(type=w1288, x=w1287) -> (*(type *) &x=w1286:refnum<vi>)
            n603 = in-place-array #121(w1286) -> (w1283:refnum<vi>[])  [unwired: 1 out]
          }
          n604 = in-place-cluster #120("Cluster_Refs"=w1283) -> (w1274:refnum<class "DIG_IO.lvclass">)
        }
      }
      frame "Bank 58" {
        n605 = String Subset(string=w1290, offset (0)=5) -> (substring=w1292:string)  [unwired: 1 in]
        n606 = Decimal String To Number(string=w1292) -> (number=w1289:i32)  [unwired: 2 in, 1 out]
        n607 = in-place {
          in-place-border: w1296 -> [w1302]
          in-place-border: w1294 -> [w1303]
          in-place-border: [w1301] -> w1293
          in-place-border: w1289 -> [w1300]
          n608 = in-place-cluster #122(w1297) -> ("Cluster_Refs"=w1305:refnum<vi>[])
          n609 = property class="Ctl"(reference=w1303, "Visible"=FALSE) -> (reference out=w1299:refnum<vi>)  [unwired: 1 in, 1 out]
          n610 = in-place {
            in-place-border: w1299 -> [w1308]
            in-place-border: w1302 -> [w1306]
            in-place-border: [w1306] -> w1301
            n611 = in-place-array #123(w1305, w1300) -> (w1309:refnum<vi>)
            n612 = Type Cast(type=w1309, x=w1308) -> (*(type *) &x=w1307:refnum<vi>)
            n613 = in-place-array #123(w1307) -> (w1304:refnum<vi>[])  [unwired: 1 out]
          }
          n614 = in-place-cluster #122("Cluster_Refs"=w1304) -> (w1295:refnum<class "DIG_IO.lvclass">)
        }
      }
      frame "Bank 59" {
        n615 = String Subset(string=w1311, offset (0)=5) -> (substring=w1313:string)  [unwired: 1 in]
        n616 = Decimal String To Number(string=w1313) -> (number=w1310:i32)  [unwired: 2 in, 1 out]
        n617 = in-place {
          in-place-border: w1317 -> [w1323]
          in-place-border: w1315 -> [w1324]
          in-place-border: [w1322] -> w1314
          in-place-border: w1310 -> [w1321]
          n618 = in-place-cluster #124(w1318) -> ("Cluster_Refs"=w1326:refnum<vi>[])
          n619 = property class="Ctl"(reference=w1324, "Visible"=FALSE) -> (reference out=w1320:refnum<vi>)  [unwired: 1 in, 1 out]
          n620 = in-place {
            in-place-border: w1320 -> [w1329]
            in-place-border: w1323 -> [w1327]
            in-place-border: [w1327] -> w1322
            n621 = in-place-array #125(w1326, w1321) -> (w1330:refnum<vi>)
            n622 = Type Cast(type=w1330, x=w1329) -> (*(type *) &x=w1328:refnum<vi>)
            n623 = in-place-array #125(w1328) -> (w1325:refnum<vi>[])  [unwired: 1 out]
          }
          n624 = in-place-cluster #124("Cluster_Refs"=w1325) -> (w1316:refnum<class "DIG_IO.lvclass">)
        }
      }
      frame "Bank 60" {
        n625 = String Subset(string=w1332, offset (0)=5) -> (substring=w1334:string)  [unwired: 1 in]
        n626 = Decimal String To Number(string=w1334) -> (number=w1331:i32)  [unwired: 2 in, 1 out]
        n627 = in-place {
          in-place-border: w1338 -> [w1344]
          in-place-border: w1336 -> [w1345]
          in-place-border: [w1343] -> w1335
          in-place-border: w1331 -> [w1342]
          n628 = in-place-cluster #126(w1339) -> ("Cluster_Refs"=w1347:refnum<vi>[])
          n629 = property class="Ctl"(reference=w1345, "Visible"=FALSE) -> (reference out=w1341:refnum<vi>)  [unwired: 1 in, 1 out]
          n630 = in-place {
            in-place-border: w1341 -> [w1350]
            in-place-border: w1344 -> [w1348]
            in-place-border: [w1348] -> w1343
            n631 = in-place-array #127(w1347, w1342) -> (w1351:refnum<vi>)
            n632 = Type Cast(type=w1351, x=w1350) -> (*(type *) &x=w1349:refnum<vi>)
            n633 = in-place-array #127(w1349) -> (w1346:refnum<vi>[])  [unwired: 1 out]
          }
          n634 = in-place-cluster #126("Cluster_Refs"=w1346) -> (w1337:refnum<class "DIG_IO.lvclass">)
        }
      }
      frame "Bank 61" {
        n635 = String Subset(string=w1353, offset (0)=5) -> (substring=w1355:string)  [unwired: 1 in]
        n636 = Decimal String To Number(string=w1355) -> (number=w1352:i32)  [unwired: 2 in, 1 out]
        n637 = in-place {
          in-place-border: w1359 -> [w1365]
          in-place-border: w1357 -> [w1366]
          in-place-border: [w1364] -> w1356
          in-place-border: w1352 -> [w1363]
          n638 = in-place-cluster #128(w1360) -> ("Cluster_Refs"=w1368:refnum<vi>[])
          n639 = property class="Ctl"(reference=w1366, "Visible"=FALSE) -> (reference out=w1362:refnum<vi>)  [unwired: 1 in, 1 out]
          n640 = in-place {
            in-place-border: w1362 -> [w1371]
            in-place-border: w1365 -> [w1369]
            in-place-border: [w1369] -> w1364
            n641 = in-place-array #129(w1368, w1363) -> (w1372:refnum<vi>)
            n642 = Type Cast(type=w1372, x=w1371) -> (*(type *) &x=w1370:refnum<vi>)
            n643 = in-place-array #129(w1370) -> (w1367:refnum<vi>[])  [unwired: 1 out]
          }
          n644 = in-place-cluster #128("Cluster_Refs"=w1367) -> (w1358:refnum<class "DIG_IO.lvclass">)
        }
      }
      frame "Bank 62" {
        n645 = String Subset(string=w1374, offset (0)=5) -> (substring=w1376:string)  [unwired: 1 in]
        n646 = Decimal String To Number(string=w1376) -> (number=w1373:i32)  [unwired: 2 in, 1 out]
        n647 = in-place {
          in-place-border: w1380 -> [w1386]
          in-place-border: w1378 -> [w1387]
          in-place-border: [w1385] -> w1377
          in-place-border: w1373 -> [w1384]
          n648 = in-place-cluster #130(w1381) -> ("Cluster_Refs"=w1389:refnum<vi>[])
          n649 = property class="Ctl"(reference=w1387, "Visible"=FALSE) -> (reference out=w1383:refnum<vi>)  [unwired: 1 in, 1 out]
          n650 = in-place {
            in-place-border: w1383 -> [w1392]
            in-place-border: w1386 -> [w1390]
            in-place-border: [w1390] -> w1385
            n651 = in-place-array #131(w1389, w1384) -> (w1393:refnum<vi>)
            n652 = Type Cast(type=w1393, x=w1392) -> (*(type *) &x=w1391:refnum<vi>)
            n653 = in-place-array #131(w1391) -> (w1388:refnum<vi>[])  [unwired: 1 out]
          }
          n654 = in-place-cluster #130("Cluster_Refs"=w1388) -> (w1379:refnum<class "DIG_IO.lvclass">)
        }
      }
      frame "Bank 63" {
        n655 = String Subset(string=w1395, offset (0)=5) -> (substring=w1397:string)  [unwired: 1 in]
        n656 = Decimal String To Number(string=w1397) -> (number=w1394:i32)  [unwired: 2 in, 1 out]
        n657 = in-place {
          in-place-border: w1401 -> [w1407]
          in-place-border: w1399 -> [w1408]
          in-place-border: [w1406] -> w1398
          in-place-border: w1394 -> [w1405]
          n658 = in-place-cluster #132(w1402) -> ("Cluster_Refs"=w1410:refnum<vi>[])
          n659 = property class="Ctl"(reference=w1408, "Visible"=FALSE) -> (reference out=w1404:refnum<vi>)  [unwired: 1 in, 1 out]
          n660 = in-place {
            in-place-border: w1404 -> [w1413]
            in-place-border: w1407 -> [w1411]
            in-place-border: [w1411] -> w1406
            n661 = in-place-array #133(w1410, w1405) -> (w1414:refnum<vi>)
            n662 = Type Cast(type=w1414, x=w1413) -> (*(type *) &x=w1412:refnum<vi>)
            n663 = in-place-array #133(w1412) -> (w1409:refnum<vi>[])  [unwired: 1 out]
          }
          n664 = in-place-cluster #132("Cluster_Refs"=w1409) -> (w1400:refnum<class "DIG_IO.lvclass">)
        }
      }
      frame "Bank 64" {
        n665 = String Subset(string=w1416, offset (0)=5) -> (substring=w1418:string)  [unwired: 1 in]
        n666 = Decimal String To Number(string=w1418) -> (number=w1415:i32)  [unwired: 2 in, 1 out]
        n667 = in-place {
          in-place-border: w1422 -> [w1428]
          in-place-border: w1420 -> [w1429]
          in-place-border: [w1427] -> w1419
          in-place-border: w1415 -> [w1426]
          n668 = in-place-cluster #134(w1423) -> ("Cluster_Refs"=w1431:refnum<vi>[])
          n669 = property class="Ctl"(reference=w1429, "Visible"=FALSE) -> (reference out=w1425:refnum<vi>)  [unwired: 1 in, 1 out]
          n670 = in-place {
            in-place-border: w1425 -> [w1434]
            in-place-border: w1428 -> [w1432]
            in-place-border: [w1432] -> w1427
            n671 = in-place-array #135(w1431, w1426) -> (w1435:refnum<vi>)
            n672 = Type Cast(type=w1435, x=w1434) -> (*(type *) &x=w1433:refnum<vi>)
            n673 = in-place-array #135(w1433) -> (w1430:refnum<vi>[])  [unwired: 1 out]
          }
          n674 = in-place-cluster #134("Cluster_Refs"=w1430) -> (w1421:refnum<class "DIG_IO.lvclass">)
        }
      }
      frame "Bank 65" {
        n675 = String Subset(string=w1437, offset (0)=5) -> (substring=w1439:string)  [unwired: 1 in]
        n676 = Decimal String To Number(string=w1439) -> (number=w1436:i32)  [unwired: 2 in, 1 out]
        n677 = in-place {
          in-place-border: w1443 -> [w1449]
          in-place-border: w1441 -> [w1450]
          in-place-border: [w1448] -> w1440
          in-place-border: w1436 -> [w1447]
          n678 = in-place-cluster #136(w1444) -> ("Cluster_Refs"=w1452:refnum<vi>[])
          n679 = property class="Ctl"(reference=w1450, "Visible"=FALSE) -> (reference out=w1446:refnum<vi>)  [unwired: 1 in, 1 out]
          n680 = in-place {
            in-place-border: w1446 -> [w1455]
            in-place-border: w1449 -> [w1453]
            in-place-border: [w1453] -> w1448
            n681 = in-place-array #137(w1452, w1447) -> (w1456:refnum<vi>)
            n682 = Type Cast(type=w1456, x=w1455) -> (*(type *) &x=w1454:refnum<vi>)
            n683 = in-place-array #137(w1454) -> (w1451:refnum<vi>[])  [unwired: 1 out]
          }
          n684 = in-place-cluster #136("Cluster_Refs"=w1451) -> (w1442:refnum<class "DIG_IO.lvclass">)
        }
      }
      frame "Bank 66" {
        n685 = String Subset(string=w1458, offset (0)=5) -> (substring=w1460:string)  [unwired: 1 in]
        n686 = Decimal String To Number(string=w1460) -> (number=w1457:i32)  [unwired: 2 in, 1 out]
        n687 = in-place {
          in-place-border: w1464 -> [w1470]
          in-place-border: w1462 -> [w1471]
          in-place-border: [w1469] -> w1461
          in-place-border: w1457 -> [w1468]
          n688 = in-place-cluster #138(w1465) -> ("Cluster_Refs"=w1473:refnum<vi>[])
          n689 = property class="Ctl"(reference=w1471, "Visible"=FALSE) -> (reference out=w1467:refnum<vi>)  [unwired: 1 in, 1 out]
          n690 = in-place {
            in-place-border: w1467 -> [w1476]
            in-place-border: w1470 -> [w1474]
            in-place-border: [w1474] -> w1469
            n691 = in-place-array #139(w1473, w1468) -> (w1477:refnum<vi>)
            n692 = Type Cast(type=w1477, x=w1476) -> (*(type *) &x=w1475:refnum<vi>)
            n693 = in-place-array #139(w1475) -> (w1472:refnum<vi>[])  [unwired: 1 out]
          }
          n694 = in-place-cluster #138("Cluster_Refs"=w1472) -> (w1463:refnum<class "DIG_IO.lvclass">)
        }
      }
      frame "Bank 67" {
        n695 = String Subset(string=w1479, offset (0)=5) -> (substring=w1481:string)  [unwired: 1 in]
        n696 = Decimal String To Number(string=w1481) -> (number=w1478:i32)  [unwired: 2 in, 1 out]
        n697 = in-place {
          in-place-border: w1485 -> [w1491]
          in-place-border: w1483 -> [w1492]
          in-place-border: [w1490] -> w1482
          in-place-border: w1478 -> [w1489]
          n698 = in-place-cluster #140(w1486) -> ("Cluster_Refs"=w1494:refnum<vi>[])
          n699 = property class="Ctl"(reference=w1492, "Visible"=FALSE) -> (reference out=w1488:refnum<vi>)  [unwired: 1 in, 1 out]
          n700 = in-place {
            in-place-border: w1488 -> [w1497]
            in-place-border: w1491 -> [w1495]
            in-place-border: [w1495] -> w1490
            n701 = in-place-array #141(w1494, w1489) -> (w1498:refnum<vi>)
            n702 = Type Cast(type=w1498, x=w1497) -> (*(type *) &x=w1496:refnum<vi>)
            n703 = in-place-array #141(w1496) -> (w1493:refnum<vi>[])  [unwired: 1 out]
          }
          n704 = in-place-cluster #140("Cluster_Refs"=w1493) -> (w1484:refnum<class "DIG_IO.lvclass">)
        }
      }
      frame "Bank 68" {
        n705 = String Subset(string=w1500, offset (0)=5) -> (substring=w1502:string)  [unwired: 1 in]
        n706 = Decimal String To Number(string=w1502) -> (number=w1499:i32)  [unwired: 2 in, 1 out]
        n707 = in-place {
          in-place-border: w1506 -> [w1512]
          in-place-border: w1504 -> [w1513]
          in-place-border: [w1511] -> w1503
          in-place-border: w1499 -> [w1510]
          n708 = in-place-cluster #142(w1507) -> ("Cluster_Refs"=w1515:refnum<vi>[])
          n709 = property class="Ctl"(reference=w1513, "Visible"=FALSE) -> (reference out=w1509:refnum<vi>)  [unwired: 1 in, 1 out]
          n710 = in-place {
            in-place-border: w1509 -> [w1518]
            in-place-border: w1512 -> [w1516]
            in-place-border: [w1516] -> w1511
            n711 = in-place-array #143(w1515, w1510) -> (w1519:refnum<vi>)
            n712 = Type Cast(type=w1519, x=w1518) -> (*(type *) &x=w1517:refnum<vi>)
            n713 = in-place-array #143(w1517) -> (w1514:refnum<vi>[])  [unwired: 1 out]
          }
          n714 = in-place-cluster #142("Cluster_Refs"=w1514) -> (w1505:refnum<class "DIG_IO.lvclass">)
        }
      }
      frame "Bank 69" {
        n715 = String Subset(string=w1521, offset (0)=5) -> (substring=w1523:string)  [unwired: 1 in]
        n716 = Decimal String To Number(string=w1523) -> (number=w1520:i32)  [unwired: 2 in, 1 out]
        n717 = in-place {
          in-place-border: w1527 -> [w1533]
          in-place-border: w1525 -> [w1534]
          in-place-border: [w1532] -> w1524
          in-place-border: w1520 -> [w1531]
          n718 = in-place-cluster #144(w1528) -> ("Cluster_Refs"=w1536:refnum<vi>[])
          n719 = property class="Ctl"(reference=w1534, "Visible"=FALSE) -> (reference out=w1530:refnum<vi>)  [unwired: 1 in, 1 out]
          n720 = in-place {
            in-place-border: w1530 -> [w1539]
            in-place-border: w1533 -> [w1537]
            in-place-border: [w1537] -> w1532
            n721 = in-place-array #145(w1536, w1531) -> (w1540:refnum<vi>)
            n722 = Type Cast(type=w1540, x=w1539) -> (*(type *) &x=w1538:refnum<vi>)
            n723 = in-place-array #145(w1538) -> (w1535:refnum<vi>[])  [unwired: 1 out]
          }
          n724 = in-place-cluster #144("Cluster_Refs"=w1535) -> (w1526:refnum<class "DIG_IO.lvclass">)
        }
      }
      frame "Bank 70" {
        n725 = String Subset(string=w1542, offset (0)=5) -> (substring=w1544:string)  [unwired: 1 in]
        n726 = Decimal String To Number(string=w1544) -> (number=w1541:i32)  [unwired: 2 in, 1 out]
        n727 = in-place {
          in-place-border: w1548 -> [w1554]
          in-place-border: w1546 -> [w1555]
          in-place-border: [w1553] -> w1545
          in-place-border: w1541 -> [w1552]
          n728 = in-place-cluster #146(w1549) -> ("Cluster_Refs"=w1557:refnum<vi>[])
          n729 = property class="Ctl"(reference=w1555, "Visible"=FALSE) -> (reference out=w1551:refnum<vi>)  [unwired: 1 in, 1 out]
          n730 = in-place {
            in-place-border: w1551 -> [w1560]
            in-place-border: w1554 -> [w1558]
            in-place-border: [w1558] -> w1553
            n731 = in-place-array #147(w1557, w1552) -> (w1561:refnum<vi>)
            n732 = Type Cast(type=w1561, x=w1560) -> (*(type *) &x=w1559:refnum<vi>)
            n733 = in-place-array #147(w1559) -> (w1556:refnum<vi>[])  [unwired: 1 out]
          }
          n734 = in-place-cluster #146("Cluster_Refs"=w1556) -> (w1547:refnum<class "DIG_IO.lvclass">)
        }
      }
      frame "Bank 71" {
        n735 = String Subset(string=w1563, offset (0)=5) -> (substring=w1565:string)  [unwired: 1 in]
        n736 = Decimal String To Number(string=w1565) -> (number=w1562:i32)  [unwired: 2 in, 1 out]
        n737 = in-place {
          in-place-border: w1569 -> [w1575]
          in-place-border: w1567 -> [w1576]
          in-place-border: [w1574] -> w1566
          in-place-border: w1562 -> [w1573]
          n738 = in-place-cluster #148(w1570) -> ("Cluster_Refs"=w1578:refnum<vi>[])
          n739 = property class="Ctl"(reference=w1576, "Visible"=FALSE) -> (reference out=w1572:refnum<vi>)  [unwired: 1 in, 1 out]
          n740 = in-place {
            in-place-border: w1572 -> [w1581]
            in-place-border: w1575 -> [w1579]
            in-place-border: [w1579] -> w1574
            n741 = in-place-array #149(w1578, w1573) -> (w1582:refnum<vi>)
            n742 = Type Cast(type=w1582, x=w1581) -> (*(type *) &x=w1580:refnum<vi>)
            n743 = in-place-array #149(w1580) -> (w1577:refnum<vi>[])  [unwired: 1 out]
          }
          n744 = in-place-cluster #148("Cluster_Refs"=w1577) -> (w1568:refnum<class "DIG_IO.lvclass">)
        }
      }
      frame "Bank 72" {
        n745 = String Subset(string=w1584, offset (0)=5) -> (substring=w1586:string)  [unwired: 1 in]
        n746 = Decimal String To Number(string=w1586) -> (number=w1583:i32)  [unwired: 2 in, 1 out]
        n747 = in-place {
          in-place-border: w1590 -> [w1596]
          in-place-border: w1588 -> [w1597]
          in-place-border: [w1595] -> w1587
          in-place-border: w1583 -> [w1594]
          n748 = in-place-cluster #150(w1591) -> ("Cluster_Refs"=w1599:refnum<vi>[])
          n749 = property class="Ctl"(reference=w1597, "Visible"=FALSE) -> (reference out=w1593:refnum<vi>)  [unwired: 1 in, 1 out]
          n750 = in-place {
            in-place-border: w1593 -> [w1602]
            in-place-border: w1596 -> [w1600]
            in-place-border: [w1600] -> w1595
            n751 = in-place-array #151(w1599, w1594) -> (w1603:refnum<vi>)
            n752 = Type Cast(type=w1603, x=w1602) -> (*(type *) &x=w1601:refnum<vi>)
            n753 = in-place-array #151(w1601) -> (w1598:refnum<vi>[])  [unwired: 1 out]
          }
          n754 = in-place-cluster #150("Cluster_Refs"=w1598) -> (w1589:refnum<class "DIG_IO.lvclass">)
        }
      }
      frame "Bank 73" {
        n755 = String Subset(string=w1605, offset (0)=5) -> (substring=w1607:string)  [unwired: 1 in]
        n756 = Decimal String To Number(string=w1607) -> (number=w1604:i32)  [unwired: 2 in, 1 out]
        n757 = in-place {
          in-place-border: w1611 -> [w1617]
          in-place-border: w1609 -> [w1618]
          in-place-border: [w1616] -> w1608
          in-place-border: w1604 -> [w1615]
          n758 = in-place-cluster #152(w1612) -> ("Cluster_Refs"=w1620:refnum<vi>[])
          n759 = property class="Ctl"(reference=w1618, "Visible"=FALSE) -> (reference out=w1614:refnum<vi>)  [unwired: 1 in, 1 out]
          n760 = in-place {
            in-place-border: w1614 -> [w1623]
            in-place-border: w1617 -> [w1621]
            in-place-border: [w1621] -> w1616
            n761 = in-place-array #153(w1620, w1615) -> (w1624:refnum<vi>)
            n762 = Type Cast(type=w1624, x=w1623) -> (*(type *) &x=w1622:refnum<vi>)
            n763 = in-place-array #153(w1622) -> (w1619:refnum<vi>[])  [unwired: 1 out]
          }
          n764 = in-place-cluster #152("Cluster_Refs"=w1619) -> (w1610:refnum<class "DIG_IO.lvclass">)
        }
      }
      frame "Bank 74" {
        n765 = String Subset(string=w1626, offset (0)=5) -> (substring=w1628:string)  [unwired: 1 in]
        n766 = Decimal String To Number(string=w1628) -> (number=w1625:i32)  [unwired: 2 in, 1 out]
        n767 = in-place {
          in-place-border: w1632 -> [w1638]
          in-place-border: w1630 -> [w1639]
          in-place-border: [w1637] -> w1629
          in-place-border: w1625 -> [w1636]
          n768 = in-place-cluster #154(w1633) -> ("Cluster_Refs"=w1641:refnum<vi>[])
          n769 = property class="Ctl"(reference=w1639, "Visible"=FALSE) -> (reference out=w1635:refnum<vi>)  [unwired: 1 in, 1 out]
          n770 = in-place {
            in-place-border: w1635 -> [w1644]
            in-place-border: w1638 -> [w1642]
            in-place-border: [w1642] -> w1637
            n771 = in-place-array #155(w1641, w1636) -> (w1645:refnum<vi>)
            n772 = Type Cast(type=w1645, x=w1644) -> (*(type *) &x=w1643:refnum<vi>)
            n773 = in-place-array #155(w1643) -> (w1640:refnum<vi>[])  [unwired: 1 out]
          }
          n774 = in-place-cluster #154("Cluster_Refs"=w1640) -> (w1631:refnum<class "DIG_IO.lvclass">)
        }
      }
      frame "Bank 75" {
        n775 = String Subset(string=w1647, offset (0)=5) -> (substring=w1649:string)  [unwired: 1 in]
        n776 = Decimal String To Number(string=w1649) -> (number=w1646:i32)  [unwired: 2 in, 1 out]
        n777 = in-place {
          in-place-border: w1653 -> [w1659]
          in-place-border: w1651 -> [w1660]
          in-place-border: [w1658] -> w1650
          in-place-border: w1646 -> [w1657]
          n778 = in-place-cluster #156(w1654) -> ("Cluster_Refs"=w1662:refnum<vi>[])
          n779 = property class="Ctl"(reference=w1660, "Visible"=FALSE) -> (reference out=w1656:refnum<vi>)  [unwired: 1 in, 1 out]
          n780 = in-place {
            in-place-border: w1656 -> [w1665]
            in-place-border: w1659 -> [w1663]
            in-place-border: [w1663] -> w1658
            n781 = in-place-array #157(w1662, w1657) -> (w1666:refnum<vi>)
            n782 = Type Cast(type=w1666, x=w1665) -> (*(type *) &x=w1664:refnum<vi>)
            n783 = in-place-array #157(w1664) -> (w1661:refnum<vi>[])  [unwired: 1 out]
          }
          n784 = in-place-cluster #156("Cluster_Refs"=w1661) -> (w1652:refnum<class "DIG_IO.lvclass">)
        }
      }
      frame "Bank 76" {
        n785 = String Subset(string=w1668, offset (0)=5) -> (substring=w1670:string)  [unwired: 1 in]
        n786 = Decimal String To Number(string=w1670) -> (number=w1667:i32)  [unwired: 2 in, 1 out]
        n787 = in-place {
          in-place-border: w1674 -> [w1680]
          in-place-border: w1672 -> [w1681]
          in-place-border: [w1679] -> w1671
          in-place-border: w1667 -> [w1678]
          n788 = in-place-cluster #158(w1675) -> ("Cluster_Refs"=w1683:refnum<vi>[])
          n789 = property class="Ctl"(reference=w1681, "Visible"=FALSE) -> (reference out=w1677:refnum<vi>)  [unwired: 1 in, 1 out]
          n790 = in-place {
            in-place-border: w1677 -> [w1686]
            in-place-border: w1680 -> [w1684]
            in-place-border: [w1684] -> w1679
            n791 = in-place-array #159(w1683, w1678) -> (w1687:refnum<vi>)
            n792 = Type Cast(type=w1687, x=w1686) -> (*(type *) &x=w1685:refnum<vi>)
            n793 = in-place-array #159(w1685) -> (w1682:refnum<vi>[])  [unwired: 1 out]
          }
          n794 = in-place-cluster #158("Cluster_Refs"=w1682) -> (w1673:refnum<class "DIG_IO.lvclass">)
        }
      }
      frame "Bank 77" {
        n795 = String Subset(string=w1689, offset (0)=5) -> (substring=w1691:string)  [unwired: 1 in]
        n796 = Decimal String To Number(string=w1691) -> (number=w1688:i32)  [unwired: 2 in, 1 out]
        n797 = in-place {
          in-place-border: w1695 -> [w1701]
          in-place-border: w1693 -> [w1702]
          in-place-border: [w1700] -> w1692
          in-place-border: w1688 -> [w1699]
          n798 = in-place-cluster #160(w1696) -> ("Cluster_Refs"=w1704:refnum<vi>[])
          n799 = property class="Ctl"(reference=w1702, "Visible"=FALSE) -> (reference out=w1698:refnum<vi>)  [unwired: 1 in, 1 out]
          n800 = in-place {
            in-place-border: w1698 -> [w1707]
            in-place-border: w1701 -> [w1705]
            in-place-border: [w1705] -> w1700
            n801 = in-place-array #161(w1704, w1699) -> (w1708:refnum<vi>)
            n802 = Type Cast(type=w1708, x=w1707) -> (*(type *) &x=w1706:refnum<vi>)
            n803 = in-place-array #161(w1706) -> (w1703:refnum<vi>[])  [unwired: 1 out]
          }
          n804 = in-place-cluster #160("Cluster_Refs"=w1703) -> (w1694:refnum<class "DIG_IO.lvclass">)
        }
      }
      frame "Bank 78" {
        n805 = String Subset(string=w1710, offset (0)=5) -> (substring=w1712:string)  [unwired: 1 in]
        n806 = Decimal String To Number(string=w1712) -> (number=w1709:i32)  [unwired: 2 in, 1 out]
        n807 = in-place {
          in-place-border: w1716 -> [w1722]
          in-place-border: w1714 -> [w1723]
          in-place-border: [w1721] -> w1713
          in-place-border: w1709 -> [w1720]
          n808 = in-place-cluster #162(w1717) -> ("Cluster_Refs"=w1725:refnum<vi>[])
          n809 = property class="Ctl"(reference=w1723, "Visible"=FALSE) -> (reference out=w1719:refnum<vi>)  [unwired: 1 in, 1 out]
          n810 = in-place {
            in-place-border: w1719 -> [w1728]
            in-place-border: w1722 -> [w1726]
            in-place-border: [w1726] -> w1721
            n811 = in-place-array #163(w1725, w1720) -> (w1729:refnum<vi>)
            n812 = Type Cast(type=w1729, x=w1728) -> (*(type *) &x=w1727:refnum<vi>)
            n813 = in-place-array #163(w1727) -> (w1724:refnum<vi>[])  [unwired: 1 out]
          }
          n814 = in-place-cluster #162("Cluster_Refs"=w1724) -> (w1715:refnum<class "DIG_IO.lvclass">)
        }
      }
      frame "Bank 79" {
        n815 = String Subset(string=w1731, offset (0)=5) -> (substring=w1733:string)  [unwired: 1 in]
        n816 = Decimal String To Number(string=w1733) -> (number=w1730:i32)  [unwired: 2 in, 1 out]
        n817 = in-place {
          in-place-border: w1737 -> [w1743]
          in-place-border: w1735 -> [w1744]
          in-place-border: [w1742] -> w1734
          in-place-border: w1730 -> [w1741]
          n818 = in-place-cluster #164(w1738) -> ("Cluster_Refs"=w1746:refnum<vi>[])
          n819 = property class="Ctl"(reference=w1744, "Visible"=FALSE) -> (reference out=w1740:refnum<vi>)  [unwired: 1 in, 1 out]
          n820 = in-place {
            in-place-border: w1740 -> [w1749]
            in-place-border: w1743 -> [w1747]
            in-place-border: [w1747] -> w1742
            n821 = in-place-array #165(w1746, w1741) -> (w1750:refnum<vi>)
            n822 = Type Cast(type=w1750, x=w1749) -> (*(type *) &x=w1748:refnum<vi>)
            n823 = in-place-array #165(w1748) -> (w1745:refnum<vi>[])  [unwired: 1 out]
          }
          n824 = in-place-cluster #164("Cluster_Refs"=w1745) -> (w1736:refnum<class "DIG_IO.lvclass">)
        }
      }
      frame "Bank 80" {
        n825 = String Subset(string=w1752, offset (0)=5) -> (substring=w1754:string)  [unwired: 1 in]
        n826 = Decimal String To Number(string=w1754) -> (number=w1751:i32)  [unwired: 2 in, 1 out]
        n827 = in-place {
          in-place-border: w1758 -> [w1764]
          in-place-border: w1756 -> [w1765]
          in-place-border: [w1763] -> w1755
          in-place-border: w1751 -> [w1762]
          n828 = in-place-cluster #166(w1759) -> ("Cluster_Refs"=w1767:refnum<vi>[])
          n829 = property class="Ctl"(reference=w1765, "Visible"=FALSE) -> (reference out=w1761:refnum<vi>)  [unwired: 1 in, 1 out]
          n830 = in-place {
            in-place-border: w1761 -> [w1770]
            in-place-border: w1764 -> [w1768]
            in-place-border: [w1768] -> w1763
            n831 = in-place-array #167(w1767, w1762) -> (w1771:refnum<vi>)
            n832 = Type Cast(type=w1771, x=w1770) -> (*(type *) &x=w1769:refnum<vi>)
            n833 = in-place-array #167(w1769) -> (w1766:refnum<vi>[])  [unwired: 1 out]
          }
          n834 = in-place-cluster #166("Cluster_Refs"=w1766) -> (w1757:refnum<class "DIG_IO.lvclass">)
        }
      }
      frame "Bank 81" {
        n835 = String Subset(string=w1773, offset (0)=5) -> (substring=w1775:string)  [unwired: 1 in]
        n836 = Decimal String To Number(string=w1775) -> (number=w1772:i32)  [unwired: 2 in, 1 out]
        n837 = in-place {
          in-place-border: w1779 -> [w1785]
          in-place-border: w1777 -> [w1786]
          in-place-border: [w1784] -> w1776
          in-place-border: w1772 -> [w1783]
          n838 = in-place-cluster #168(w1780) -> ("Cluster_Refs"=w1788:refnum<vi>[])
          n839 = property class="Ctl"(reference=w1786, "Visible"=FALSE) -> (reference out=w1782:refnum<vi>)  [unwired: 1 in, 1 out]
          n840 = in-place {
            in-place-border: w1782 -> [w1791]
            in-place-border: w1785 -> [w1789]
            in-place-border: [w1789] -> w1784
            n841 = in-place-array #169(w1788, w1783) -> (w1792:refnum<vi>)
            n842 = Type Cast(type=w1792, x=w1791) -> (*(type *) &x=w1790:refnum<vi>)
            n843 = in-place-array #169(w1790) -> (w1787:refnum<vi>[])  [unwired: 1 out]
          }
          n844 = in-place-cluster #168("Cluster_Refs"=w1787) -> (w1778:refnum<class "DIG_IO.lvclass">)
        }
      }
      frame "Bank 82" {
        n845 = String Subset(string=w1794, offset (0)=5) -> (substring=w1796:string)  [unwired: 1 in]
        n846 = Decimal String To Number(string=w1796) -> (number=w1793:i32)  [unwired: 2 in, 1 out]
        n847 = in-place {
          in-place-border: w1800 -> [w1806]
          in-place-border: w1798 -> [w1807]
          in-place-border: [w1805] -> w1797
          in-place-border: w1793 -> [w1804]
          n848 = in-place-cluster #170(w1801) -> ("Cluster_Refs"=w1809:refnum<vi>[])
          n849 = property class="Ctl"(reference=w1807, "Visible"=FALSE) -> (reference out=w1803:refnum<vi>)  [unwired: 1 in, 1 out]
          n850 = in-place {
            in-place-border: w1803 -> [w1812]
            in-place-border: w1806 -> [w1810]
            in-place-border: [w1810] -> w1805
            n851 = in-place-array #171(w1809, w1804) -> (w1813:refnum<vi>)
            n852 = Type Cast(type=w1813, x=w1812) -> (*(type *) &x=w1811:refnum<vi>)
            n853 = in-place-array #171(w1811) -> (w1808:refnum<vi>[])  [unwired: 1 out]
          }
          n854 = in-place-cluster #170("Cluster_Refs"=w1808) -> (w1799:refnum<class "DIG_IO.lvclass">)
        }
      }
      frame "Bank 83" {
        n855 = String Subset(string=w1815, offset (0)=5) -> (substring=w1817:string)  [unwired: 1 in]
        n856 = Decimal String To Number(string=w1817) -> (number=w1814:i32)  [unwired: 2 in, 1 out]
        n857 = in-place {
          in-place-border: w1821 -> [w1827]
          in-place-border: w1819 -> [w1828]
          in-place-border: [w1826] -> w1818
          in-place-border: w1814 -> [w1825]
          n858 = in-place-cluster #172(w1822) -> ("Cluster_Refs"=w1830:refnum<vi>[])
          n859 = property class="Ctl"(reference=w1828, "Visible"=FALSE) -> (reference out=w1824:refnum<vi>)  [unwired: 1 in, 1 out]
          n860 = in-place {
            in-place-border: w1824 -> [w1833]
            in-place-border: w1827 -> [w1831]
            in-place-border: [w1831] -> w1826
            n861 = in-place-array #173(w1830, w1825) -> (w1834:refnum<vi>)
            n862 = Type Cast(type=w1834, x=w1833) -> (*(type *) &x=w1832:refnum<vi>)
            n863 = in-place-array #173(w1832) -> (w1829:refnum<vi>[])  [unwired: 1 out]
          }
          n864 = in-place-cluster #172("Cluster_Refs"=w1829) -> (w1820:refnum<class "DIG_IO.lvclass">)
        }
      }
      frame "Bank 84" {
        n865 = String Subset(string=w1836, offset (0)=5) -> (substring=w1838:string)  [unwired: 1 in]
        n866 = Decimal String To Number(string=w1838) -> (number=w1835:i32)  [unwired: 2 in, 1 out]
        n867 = in-place {
          in-place-border: w1842 -> [w1848]
          in-place-border: w1840 -> [w1849]
          in-place-border: [w1847] -> w1839
          in-place-border: w1835 -> [w1846]
          n868 = in-place-cluster #174(w1843) -> ("Cluster_Refs"=w1851:refnum<vi>[])
          n869 = property class="Ctl"(reference=w1849, "Visible"=FALSE) -> (reference out=w1845:refnum<vi>)  [unwired: 1 in, 1 out]
          n870 = in-place {
            in-place-border: w1845 -> [w1854]
            in-place-border: w1848 -> [w1852]
            in-place-border: [w1852] -> w1847
            n871 = in-place-array #175(w1851, w1846) -> (w1855:refnum<vi>)
            n872 = Type Cast(type=w1855, x=w1854) -> (*(type *) &x=w1853:refnum<vi>)
            n873 = in-place-array #175(w1853) -> (w1850:refnum<vi>[])  [unwired: 1 out]
          }
          n874 = in-place-cluster #174("Cluster_Refs"=w1850) -> (w1841:refnum<class "DIG_IO.lvclass">)
        }
      }
      frame "Bank 85" {
        n875 = String Subset(string=w1857, offset (0)=5) -> (substring=w1859:string)  [unwired: 1 in]
        n876 = Decimal String To Number(string=w1859) -> (number=w1856:i32)  [unwired: 2 in, 1 out]
        n877 = in-place {
          in-place-border: w1863 -> [w1869]
          in-place-border: w1861 -> [w1870]
          in-place-border: [w1868] -> w1860
          in-place-border: w1856 -> [w1867]
          n878 = in-place-cluster #176(w1864) -> ("Cluster_Refs"=w1872:refnum<vi>[])
          n879 = property class="Ctl"(reference=w1870, "Visible"=FALSE) -> (reference out=w1866:refnum<vi>)  [unwired: 1 in, 1 out]
          n880 = in-place {
            in-place-border: w1866 -> [w1875]
            in-place-border: w1869 -> [w1873]
            in-place-border: [w1873] -> w1868
            n881 = in-place-array #177(w1872, w1867) -> (w1876:refnum<vi>)
            n882 = Type Cast(type=w1876, x=w1875) -> (*(type *) &x=w1874:refnum<vi>)
            n883 = in-place-array #177(w1874) -> (w1871:refnum<vi>[])  [unwired: 1 out]
          }
          n884 = in-place-cluster #176("Cluster_Refs"=w1871) -> (w1862:refnum<class "DIG_IO.lvclass">)
        }
      }
      frame "Bank 86" {
        n885 = String Subset(string=w1878, offset (0)=5) -> (substring=w1880:string)  [unwired: 1 in]
        n886 = Decimal String To Number(string=w1880) -> (number=w1877:i32)  [unwired: 2 in, 1 out]
        n887 = in-place {
          in-place-border: w1884 -> [w1890]
          in-place-border: w1882 -> [w1891]
          in-place-border: [w1889] -> w1881
          in-place-border: w1877 -> [w1888]
          n888 = in-place-cluster #178(w1885) -> ("Cluster_Refs"=w1893:refnum<vi>[])
          n889 = property class="Ctl"(reference=w1891, "Visible"=FALSE) -> (reference out=w1887:refnum<vi>)  [unwired: 1 in, 1 out]
          n890 = in-place {
            in-place-border: w1887 -> [w1896]
            in-place-border: w1890 -> [w1894]
            in-place-border: [w1894] -> w1889
            n891 = in-place-array #179(w1893, w1888) -> (w1897:refnum<vi>)
            n892 = Type Cast(type=w1897, x=w1896) -> (*(type *) &x=w1895:refnum<vi>)
            n893 = in-place-array #179(w1895) -> (w1892:refnum<vi>[])  [unwired: 1 out]
          }
          n894 = in-place-cluster #178("Cluster_Refs"=w1892) -> (w1883:refnum<class "DIG_IO.lvclass">)
        }
      }
      frame "Bank 87" {
        n895 = String Subset(string=w1899, offset (0)=5) -> (substring=w1901:string)  [unwired: 1 in]
        n896 = Decimal String To Number(string=w1901) -> (number=w1898:i32)  [unwired: 2 in, 1 out]
        n897 = in-place {
          in-place-border: w1905 -> [w1911]
          in-place-border: w1903 -> [w1912]
          in-place-border: [w1910] -> w1902
          in-place-border: w1898 -> [w1909]
          n898 = in-place-cluster #180(w1906) -> ("Cluster_Refs"=w1914:refnum<vi>[])
          n899 = property class="Ctl"(reference=w1912, "Visible"=FALSE) -> (reference out=w1908:refnum<vi>)  [unwired: 1 in, 1 out]
          n900 = in-place {
            in-place-border: w1908 -> [w1917]
            in-place-border: w1911 -> [w1915]
            in-place-border: [w1915] -> w1910
            n901 = in-place-array #181(w1914, w1909) -> (w1918:refnum<vi>)
            n902 = Type Cast(type=w1918, x=w1917) -> (*(type *) &x=w1916:refnum<vi>)
            n903 = in-place-array #181(w1916) -> (w1913:refnum<vi>[])  [unwired: 1 out]
          }
          n904 = in-place-cluster #180("Cluster_Refs"=w1913) -> (w1904:refnum<class "DIG_IO.lvclass">)
        }
      }
      frame "Bank 88" {
        n905 = String Subset(string=w1920, offset (0)=5) -> (substring=w1922:string)  [unwired: 1 in]
        n906 = Decimal String To Number(string=w1922) -> (number=w1919:i32)  [unwired: 2 in, 1 out]
        n907 = in-place {
          in-place-border: w1926 -> [w1932]
          in-place-border: w1924 -> [w1933]
          in-place-border: [w1931] -> w1923
          in-place-border: w1919 -> [w1930]
          n908 = in-place-cluster #182(w1927) -> ("Cluster_Refs"=w1935:refnum<vi>[])
          n909 = property class="Ctl"(reference=w1933, "Visible"=FALSE) -> (reference out=w1929:refnum<vi>)  [unwired: 1 in, 1 out]
          n910 = in-place {
            in-place-border: w1929 -> [w1938]
            in-place-border: w1932 -> [w1936]
            in-place-border: [w1936] -> w1931
            n911 = in-place-array #183(w1935, w1930) -> (w1939:refnum<vi>)
            n912 = Type Cast(type=w1939, x=w1938) -> (*(type *) &x=w1937:refnum<vi>)
            n913 = in-place-array #183(w1937) -> (w1934:refnum<vi>[])  [unwired: 1 out]
          }
          n914 = in-place-cluster #182("Cluster_Refs"=w1934) -> (w1925:refnum<class "DIG_IO.lvclass">)
        }
      }
      frame "Bank 89" {
        n915 = String Subset(string=w1941, offset (0)=5) -> (substring=w1943:string)  [unwired: 1 in]
        n916 = Decimal String To Number(string=w1943) -> (number=w1940:i32)  [unwired: 2 in, 1 out]
        n917 = in-place {
          in-place-border: w1947 -> [w1953]
          in-place-border: w1945 -> [w1954]
          in-place-border: [w1952] -> w1944
          in-place-border: w1940 -> [w1951]
          n918 = in-place-cluster #184(w1948) -> ("Cluster_Refs"=w1956:refnum<vi>[])
          n919 = property class="Ctl"(reference=w1954, "Visible"=FALSE) -> (reference out=w1950:refnum<vi>)  [unwired: 1 in, 1 out]
          n920 = in-place {
            in-place-border: w1950 -> [w1959]
            in-place-border: w1953 -> [w1957]
            in-place-border: [w1957] -> w1952
            n921 = in-place-array #185(w1956, w1951) -> (w1960:refnum<vi>)
            n922 = Type Cast(type=w1960, x=w1959) -> (*(type *) &x=w1958:refnum<vi>)
            n923 = in-place-array #185(w1958) -> (w1955:refnum<vi>[])  [unwired: 1 out]
          }
          n924 = in-place-cluster #184("Cluster_Refs"=w1955) -> (w1946:refnum<class "DIG_IO.lvclass">)
        }
      }
      frame "Bank 90" {
        n925 = String Subset(string=w1962, offset (0)=5) -> (substring=w1964:string)  [unwired: 1 in]
        n926 = Decimal String To Number(string=w1964) -> (number=w1961:i32)  [unwired: 2 in, 1 out]
        n927 = in-place {
          in-place-border: w1968 -> [w1974]
          in-place-border: w1966 -> [w1975]
          in-place-border: [w1973] -> w1965
          in-place-border: w1961 -> [w1972]
          n928 = in-place-cluster #186(w1969) -> ("Cluster_Refs"=w1977:refnum<vi>[])
          n929 = property class="Ctl"(reference=w1975, "Visible"=FALSE) -> (reference out=w1971:refnum<vi>)  [unwired: 1 in, 1 out]
          n930 = in-place {
            in-place-border: w1971 -> [w1980]
            in-place-border: w1974 -> [w1978]
            in-place-border: [w1978] -> w1973
            n931 = in-place-array #187(w1977, w1972) -> (w1981:refnum<vi>)
            n932 = Type Cast(type=w1981, x=w1980) -> (*(type *) &x=w1979:refnum<vi>)
            n933 = in-place-array #187(w1979) -> (w1976:refnum<vi>[])  [unwired: 1 out]
          }
          n934 = in-place-cluster #186("Cluster_Refs"=w1976) -> (w1967:refnum<class "DIG_IO.lvclass">)
        }
      }
      frame "Bank 91" {
        n935 = String Subset(string=w1983, offset (0)=5) -> (substring=w1985:string)  [unwired: 1 in]
        n936 = Decimal String To Number(string=w1985) -> (number=w1982:i32)  [unwired: 2 in, 1 out]
        n937 = in-place {
          in-place-border: w1989 -> [w1995]
          in-place-border: w1987 -> [w1996]
          in-place-border: [w1994] -> w1986
          in-place-border: w1982 -> [w1993]
          n938 = in-place-cluster #188(w1990) -> ("Cluster_Refs"=w1998:refnum<vi>[])
          n939 = property class="Ctl"(reference=w1996, "Visible"=FALSE) -> (reference out=w1992:refnum<vi>)  [unwired: 1 in, 1 out]
          n940 = in-place {
            in-place-border: w1992 -> [w2001]
            in-place-border: w1995 -> [w1999]
            in-place-border: [w1999] -> w1994
            n941 = in-place-array #189(w1998, w1993) -> (w2002:refnum<vi>)
            n942 = Type Cast(type=w2002, x=w2001) -> (*(type *) &x=w2000:refnum<vi>)
            n943 = in-place-array #189(w2000) -> (w1997:refnum<vi>[])  [unwired: 1 out]
          }
          n944 = in-place-cluster #188("Cluster_Refs"=w1997) -> (w1988:refnum<class "DIG_IO.lvclass">)
        }
      }
      frame "Bank 92" {
        n945 = String Subset(string=w2004, offset (0)=5) -> (substring=w2006:string)  [unwired: 1 in]
        n946 = Decimal String To Number(string=w2006) -> (number=w2003:i32)  [unwired: 2 in, 1 out]
        n947 = in-place {
          in-place-border: w2010 -> [w2016]
          in-place-border: w2008 -> [w2017]
          in-place-border: [w2015] -> w2007
          in-place-border: w2003 -> [w2014]
          n948 = in-place-cluster #190(w2011) -> ("Cluster_Refs"=w2019:refnum<vi>[])
          n949 = property class="Ctl"(reference=w2017, "Visible"=FALSE) -> (reference out=w2013:refnum<vi>)  [unwired: 1 in, 1 out]
          n950 = in-place {
            in-place-border: w2013 -> [w2022]
            in-place-border: w2016 -> [w2020]
            in-place-border: [w2020] -> w2015
            n951 = in-place-array #191(w2019, w2014) -> (w2023:refnum<vi>)
            n952 = Type Cast(type=w2023, x=w2022) -> (*(type *) &x=w2021:refnum<vi>)
            n953 = in-place-array #191(w2021) -> (w2018:refnum<vi>[])  [unwired: 1 out]
          }
          n954 = in-place-cluster #190("Cluster_Refs"=w2018) -> (w2009:refnum<class "DIG_IO.lvclass">)
        }
      }
      frame "Bank 93" {
        n955 = String Subset(string=w2025, offset (0)=5) -> (substring=w2027:string)  [unwired: 1 in]
        n956 = Decimal String To Number(string=w2027) -> (number=w2024:i32)  [unwired: 2 in, 1 out]
        n957 = in-place {
          in-place-border: w2031 -> [w2037]
          in-place-border: w2029 -> [w2038]
          in-place-border: [w2036] -> w2028
          in-place-border: w2024 -> [w2035]
          n958 = in-place-cluster #192(w2032) -> ("Cluster_Refs"=w2040:refnum<vi>[])
          n959 = property class="Ctl"(reference=w2038, "Visible"=FALSE) -> (reference out=w2034:refnum<vi>)  [unwired: 1 in, 1 out]
          n960 = in-place {
            in-place-border: w2034 -> [w2043]
            in-place-border: w2037 -> [w2041]
            in-place-border: [w2041] -> w2036
            n961 = in-place-array #193(w2040, w2035) -> (w2044:refnum<vi>)
            n962 = Type Cast(type=w2044, x=w2043) -> (*(type *) &x=w2042:refnum<vi>)
            n963 = in-place-array #193(w2042) -> (w2039:refnum<vi>[])  [unwired: 1 out]
          }
          n964 = in-place-cluster #192("Cluster_Refs"=w2039) -> (w2030:refnum<class "DIG_IO.lvclass">)
        }
      }
      frame "Bank 94" {
        n965 = String Subset(string=w2046, offset (0)=5) -> (substring=w2048:string)  [unwired: 1 in]
        n966 = Decimal String To Number(string=w2048) -> (number=w2045:i32)  [unwired: 2 in, 1 out]
        n967 = in-place {
          in-place-border: w2052 -> [w2058]
          in-place-border: w2050 -> [w2059]
          in-place-border: [w2057] -> w2049
          in-place-border: w2045 -> [w2056]
          n968 = in-place-cluster #194(w2053) -> ("Cluster_Refs"=w2061:refnum<vi>[])
          n969 = property class="Ctl"(reference=w2059, "Visible"=FALSE) -> (reference out=w2055:refnum<vi>)  [unwired: 1 in, 1 out]
          n970 = in-place {
            in-place-border: w2055 -> [w2064]
            in-place-border: w2058 -> [w2062]
            in-place-border: [w2062] -> w2057
            n971 = in-place-array #195(w2061, w2056) -> (w2065:refnum<vi>)
            n972 = Type Cast(type=w2065, x=w2064) -> (*(type *) &x=w2063:refnum<vi>)
            n973 = in-place-array #195(w2063) -> (w2060:refnum<vi>[])  [unwired: 1 out]
          }
          n974 = in-place-cluster #194("Cluster_Refs"=w2060) -> (w2051:refnum<class "DIG_IO.lvclass">)
        }
      }
      frame "Bank 95" {
        n975 = String Subset(string=w2067, offset (0)=5) -> (substring=w2069:string)  [unwired: 1 in]
        n976 = Decimal String To Number(string=w2069) -> (number=w2066:i32)  [unwired: 2 in, 1 out]
        n977 = in-place {
          in-place-border: w2073 -> [w2079]
          in-place-border: w2071 -> [w2080]
          in-place-border: [w2078] -> w2070
          in-place-border: w2066 -> [w2077]
          n978 = in-place-cluster #196(w2074) -> ("Cluster_Refs"=w2082:refnum<vi>[])
          n979 = property class="Ctl"(reference=w2080, "Visible"=FALSE) -> (reference out=w2076:refnum<vi>)  [unwired: 1 in, 1 out]
          n980 = in-place {
            in-place-border: w2076 -> [w2085]
            in-place-border: w2079 -> [w2083]
            in-place-border: [w2083] -> w2078
            n981 = in-place-array #197(w2082, w2077) -> (w2086:refnum<vi>)
            n982 = Type Cast(type=w2086, x=w2085) -> (*(type *) &x=w2084:refnum<vi>)
            n983 = in-place-array #197(w2084) -> (w2081:refnum<vi>[])  [unwired: 1 out]
          }
          n984 = in-place-cluster #196("Cluster_Refs"=w2081) -> (w2072:refnum<class "DIG_IO.lvclass">)
        }
      }
      frame "QueryCurrent" {
        n985 = String Subset(string=w2088, offset (0)=5) -> (substring=w2090:string)  [unwired: 1 in]
        n986 = Decimal String To Number(string=w2090) -> (number=w2087:i32)  [unwired: 2 in, 1 out]
        n987 = in-place {
          in-place-border: w2094 -> [w2100]
          in-place-border: w2092 -> [w2101]
          in-place-border: [w2100] -> w2091
          in-place-border: w2087 -> [_]
          n988 = in-place-cluster #198(w2095) -> ("Current_Query_ref"=w2098:refnum<vi>)
          n989 = property class="Ctl"(reference=w2101, "Visible"=FALSE) -> (reference out=w2097:refnum<vi>)  [unwired: 1 in, 1 out]
          n990 = Type Cast(type=w2098, x=w2097) -> (*(type *) &x=w2096:refnum<vi>)
          n991 = in-place-cluster #198("Current_Query_ref"=w2096) -> (w2093:refnum<class "DIG_IO.lvclass">)
        }
      }
      frame "Detected Current" {
        n992 = String Subset(string=w2103, offset (0)=5) -> (substring=w2105:string)  [unwired: 1 in]
        n993 = Decimal String To Number(string=w2105) -> (number=w2102:i32)  [unwired: 2 in, 1 out]
        n994 = in-place {
          in-place-border: w2109 -> [w2115]
          in-place-border: w2107 -> [w2116]
          in-place-border: [w2115] -> w2106
          in-place-border: w2102 -> [_]
          n995 = in-place-cluster #199(w2110) -> ("Detected_Current_ref"=w2113:refnum<vi>)
          n996 = property class="Ctl"(reference=w2116, "Visible"=FALSE) -> (reference out=w2112:refnum<vi>)  [unwired: 1 in, 1 out]
          n997 = Type Cast(type=w2113, x=w2112) -> (*(type *) &x=w2111:refnum<vi>)
          n998 = in-place-cluster #199("Detected_Current_ref"=w2111) -> (w2108:refnum<class "DIG_IO.lvclass">)
        }
      }
    }
  }
  n999 = call-parent "Link Control References.vi"("error in (no error)"=w3, "Control Map"=w5, "Instruments in"=w1) -> ("error out"=→"error out":errorcluster, "Instruments out"=→"DIG_IO out":refnum<class "DIG_IO.lvclass">)  [unwired: 7 in]
